vi "Scan Module.vi"(9 "Init state":T1=enum."Init(GPU FFT)", 11 "Error In":errorcluster, 12 "Start Acquire?":bool) -> (4 "Finished?":bool, 15 "Error Out":errorcluster)   [LabVIEW 2018]
uses:
  Controls/Go Scan Actions.ctl
  Controls/Queue Manager Actions.ctl
  Controls/FGV Actions.ctl
  Controls/Set Get Controls.ctl
  Hardware Mfg/Thorlabs Translation Stages/Controls/Motion Translation Module Control2.ctl
  Tile naming actions.ctl
  Controls/scan status.ctl
  Hardware Mfg/AlazarTech SDK/Controls/Alazar Engine Actions.ctl
  type defines/Pause action.ctl
  Controls/file variable action.ctl
  Controls/vibratome3 control.ctl
  Controls/Save Bline to Mem Control.ctl
  Hardware Mfg/Thorlabs Translation Stages/Controls/Motion Translation Module Control.ctl
panel:
  in  "No Slice?":bool
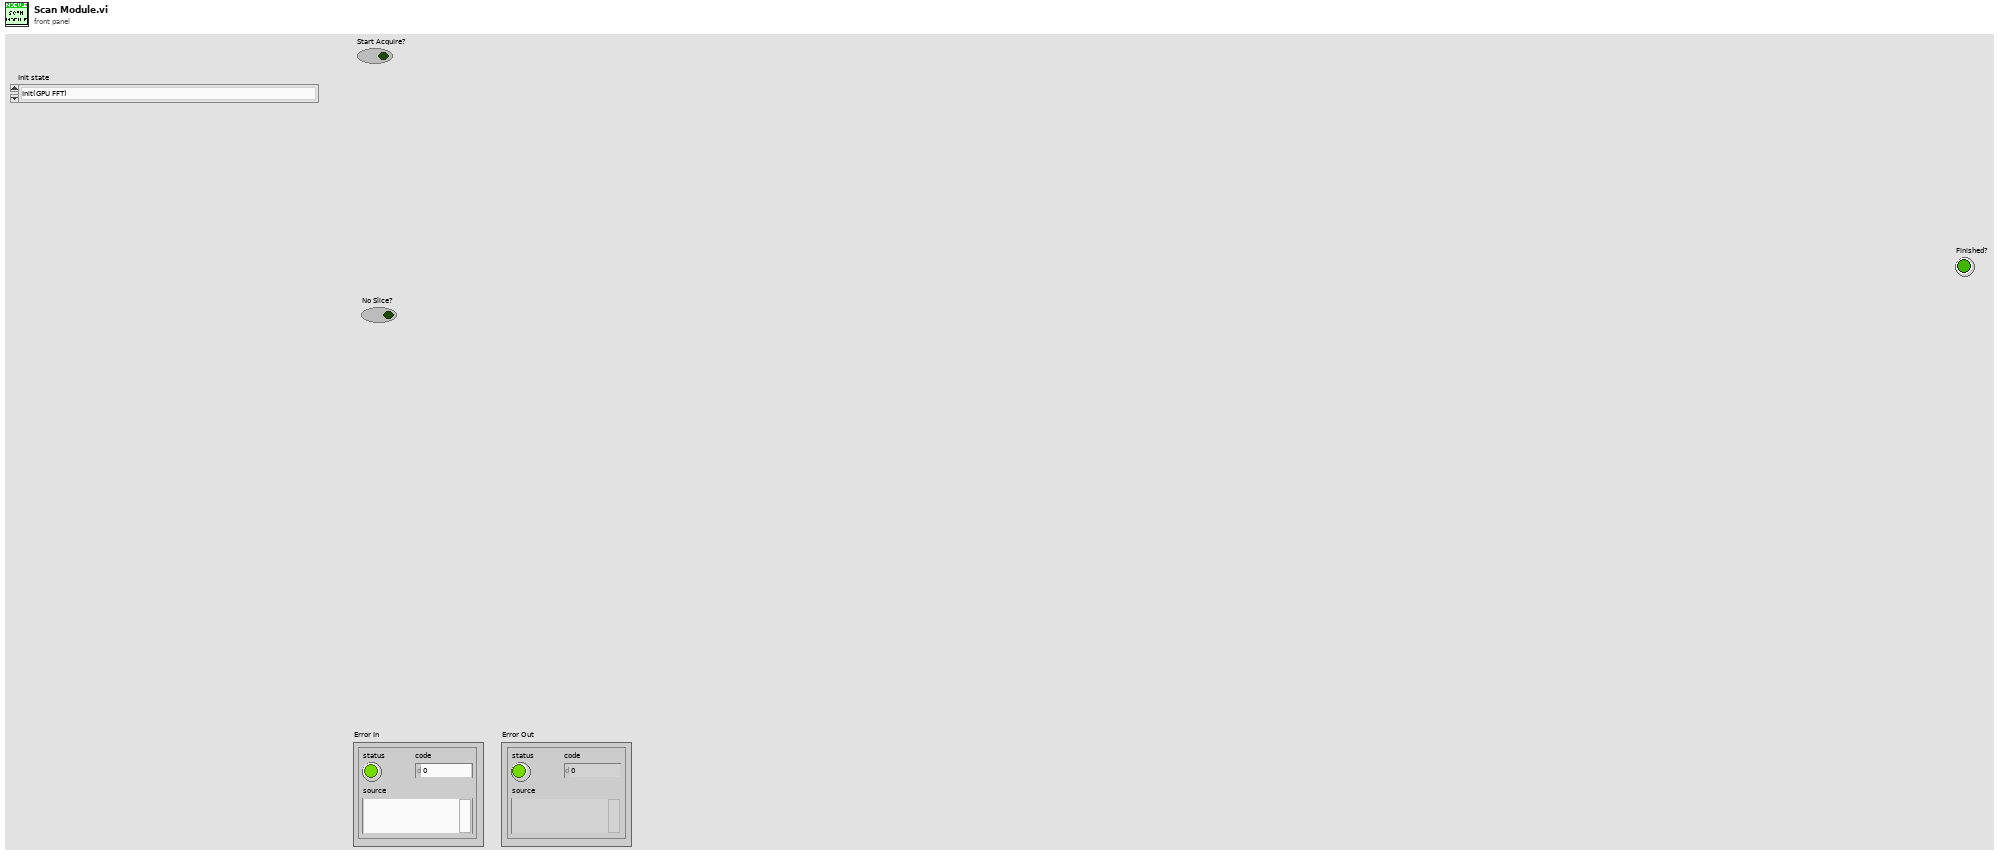
[diagram p1: front panel]
types:
  T1 = typedef "Go Scan Actions.ctl" = enum16{"Init(ThorOCT Spatial)", "Init(ThorOCT Spectral)", "Init(GPU FFT)", "Init(Alazar FFT)", "Init Scan Head(ThorOCT Spectral)", "Init Scan Head(ThorOCT Spatial)", "Init Scan Head", "Init Table Stage", "Init Vibratome", "Generate Mosaic", "Generate Z Position", "Go to Image Z", "Go Image Home", "Go Mosaic", "Acquire Image(ThorOCT Spatial)", "Acquire Image(ThorOCT Spectral)", "Acquire Image(GPU FFT)", "Acquire Image(Alazar FFT)", "Go Vibratome", "Slice", "Finished(ThorOCT)", "Finished", "Init(Alazar Spectral)", "Go Vibratome3"}
  T2 = typedef "Queue Manager Actions.ctl" = enum16{"Init", "Enqueue", "Enqueue All", "Preview Queue", "Dequeue", "Get Status", "Flush Queue", "Flush All Queues", "Release All Queues", "Release Queue", "Enqueue at Opposite End"}
  T3 = typedef "FGV Actions.ctl" = enum16{"Init", "Set", "Get", "Clear"}
  T4 = typedef "Motion Translation Module Control2.ctl" = enum16{"Init", "Home", "Status", "Velocity/Accel", "Position", "Jog", "Stop", "Uninit", "Enable", "Disable"}
  T5 = typedef "Set Get Controls.ctl" = enum16{"Set", "Get"}
  T6 = typedef "Motion Translation Module Control.ctl" = enum16{"Init", "Home", "Status", "Velocity/Accel", "Position", "Jog", "Stop", "Uninit", "Enable", "Disable"}
  T7 = typedef "Tile naming actions.ctl" = enum16{"Export", "Increment", "Total tile num", "Init"}
  T8 = typedef "scan status.ctl" = enum16{"Complete Scan(ThorOCT)", "Complete Scan(PSOCT)", "Start(ThorOCT Spatial)", "Start(ThorOCT Spectral)", "Start(GPU FFT)", "Start(Alazar FFT)", "Scan(ThorOCT Spatial)", "Scan(ThorOCT Spectral)", "Scan(GPU FFT)", "Scan(Alazar FFT)", "Finish Scan(ThorOCT)", "Finish Scan(PSOCT)", "Scan(simulate)", "Start(ROI)"}
  T9 = typedef "Alazar Engine Actions.ctl" = enum16{"Init", "Config Clock", "Config Ch", "Config Trig", "Config Non-FFT Acq.", "Non-FFT Acquire", "start acquire", "Config Acq.", "Acquire", "UnInit"}
  T10 = enum16{"Configure channels", "Write Scan Pattern", "Start Galvo Task", "Is Task Done?", "Stop Galvo", "Uninit", "Init: Calc scan pattern"}
  T11 = typedef "Pause action.ctl" = enum16{"Init", "get", "set"}
  T12 = typedef "file variable action.ctl" = enum16{"File name", "X stage", "Y stage", "Slice plane", "Image plane", "time", "output", "Init", "Memory Usage", "Disk full Space", "Disk free space"}
  T13 = typedef "vibratome3 control.ctl" = enum16{"Init", "Configure channel", "Write waveform", "Start", "Stop", "Finish?", "Uninit"}
  T14 = typedef "Save Bline to Mem Control.ctl" = enum16{"Output data", "Save(ThorOCT)", "Save(PSOCT)", "FFT and Save", "Uninit", "PSOCT Spectral buffer Set", "PSOCT Spatial buffer Set", "PSOCT Spectral buffer Init", "PSOCT Spatial buffer Init", "ThorOCT Spectral buffer Init", "ThorOCT Spatial buffer Init", "ThorOCT Spectral buffer Set", "ThorOCT Spatial buffer Set", "ThorOCT Spectral Save", "Alazar Spectral Save", "PSOCT save all"}
  T15 = typedef "ScanType.ctl" = enum16{"Single Frame", "Continuous Frame", "ROI Line", "Vibratome", "Mosaic", "Mosaic + Slice"}
  T16 = typedef "System Parameters.ctl" = cluster{"Optical Parameters":T17, "Vibratome":T18, "Table Stages":T19, "Imaging Parameter":T22, "Galvo HW Parameters":cluster{"Analog Out Channel":tag, "Min Voltage":dbl, "Max Voltage":dbl, "Pixel Clock Source":tag, "Sample Rate":dbl, "Line Clock Out Ch":tag}, "Alazar parameters":T24, "Mosaic Paramter":cluster{"X Axis":cluster{"Start [mm]":dbl, "Steps [pts]":dbl, "End [mm]":dbl}, "Y Axis":cluster{"Start [mm]":dbl, "Steps [pts]":dbl, "End [mm]":dbl}, "Scan Pattern":enum16{"Uni-directional", "Bi-Directional", "Spiral Out", "Spiral In"}, "Overlap Options":cluster{"Overlap Type":enum16{"No Overlap", "X Only", "Y Only", "X and Y"}, "Percent Overlap":u8, "Justify":enum16{"Start", "Center", "End"}}}, "Manual Controls":T31, "Vibratome Axis":T34}
  T17 = typedef "Optical Parameters.ctl" = cluster{"Obj. Focal Length [mm]":dbl, "Scan Lens EFL[mm]":dbl, "Tube Lens EFL[mm]":dbl, "Galvo V Range (+/-)":dbl, "Galvo Max Half Angle [Deg]":dbl, "Max Galvo Range[%]":dbl}
  T18 = typedef "Vibratome Parameters.ctl" = cluster{"Z Bottom [mm]":dbl, "Pre Cut Dwell [s]":dbl, "Blade Frequency [RPM]":u16, "Slice Speed [mm/s]":dbl, "Post Cut Dwell [s]":dbl, "Ramp Time [s]":dbl, "Start X [mm]":dbl, "Start Y [mm]":dbl, "Slice Length [mm]":dbl, "Slice Axis":enum16{"X Axis", "Y Axis", "Z Axis"}, "Controller VISA Ref":refnum<visa-resource-name>, "Blade Frequency [Hz]":u16, "Analog Out Channel":tag, "Pixel Clock Source":tag}
  T19 = typedef "Translation Stage Parameters.ctl" = cluster{"X Stage":T20, "Y Stage":T20, "Z Stage":T20}
  T20 = typedef "Translation Stage Cluster.ctl" = cluster{"Position":dbl, "Is.Enabled?":bool, "Is.Connected?":bool, "Device SN":string, "AccelerationMaximum":dbl, "VelocityMaximum":dbl, "Acceleration":dbl, "Velocity":dbl, "waitTimeout (ms)":i32, "Model":T21, "Is.Homed?":bool, "MOVE":bool}
  T21 = typedef "Translation Stage Types.ctl" = enum16{"None", "Thorlabs LTS", "Thorlabs MLJ"}
  T22 = typedef "Imaging Parameters.ctl" = cluster{"Raster Scan Direction":T23, "Pixel Dwell Time [Clock Cycles]":u16, "Flyback Time [Clock Cycles]":u16, "XY Center [um]":cluster{"X":dbl, "Y":dbl}, "Pixel Step Size [um] X":dbl, "XY Image Size":enum16{"32 x 32", "64 x 64", "128 x 128", "256 x 256", "512 x 512", "1024 x 1024", "2048 x 2048"}, "Custom":bool, "Custom Size":cluster{"X":u16, "Y":u16}, "Line Averages":u8, "Pixel Step Size [um] Y":dbl}
  T23 = typedef "Scan Direction.ctl" = enum16{"Uni Directional", "Bi Directional", "None"}
  T24 = typedef "Alazar parameters.ctl" = cluster{"Trigger Settings":cluster{"General Trigger Settings":T25, "Trigger Engine 1":T26, "Trigger Engine 2":T26}, "Device ID":T27, "Ch A Input Control":T28, "Ch B Input Control":T28, "Acq Settings":T29, "Capture Clock":T30}
  T25 = typedef "General Trigger Settings.ctl" = cluster{"Trigger Operation":u32, "Coupling ID":u32, "Range ID":u32, "Delay":u32, "Timeout Ticks":u32, "Mode":u32, "Parameter":u32}
  T26 = typedef "Trigger Engine Controls.ctl" = cluster{"Trigger Engine":u32, "Source":u32, "Slope":u32, "Level":u32}
  T27 = typedef "Alazar Device ID.ctl" = cluster{"System ID":u32, "Board ID":u32}
  T28 = typedef "Channel Input Controls.ctl" = cluster{"Channel":u8, "Coupling":u32, "Range":u32, "Impedance":u32}
  T29 = typedef "Alazar Acquisition Settings.ctl" = cluster{"Record Length":u32, "Offset":u32, "Records Per Buffer":u32, "Records Count (Records/Acq)":u32, "Window Type":u32, "Footer":u32, "Samples per record":u32, "Output Format":u32}
  T30 = typedef "Clock Controls.ctl" = cluster{"Sample Rate":u32, "Decimation":u32, "Source":u32, "Edge":u32}
  T31 = typedef "Manual Controls.ctl" = cluster{"Z0":dbl, "First image height":dbl, "Data Path":path, "Save parameters":T32, "Center Galvos":bool, "Acquisition mode":T33, "PSOCT Channel":u32, "Save":bool, "AIP rotation angle":dbl, "ret ds":bool, "Pause?":bool, "Outgoing Mail Server (SMTP)":string, "Email":string, "Password":string, "Carrier 1":enum16{"T-Mobile", "AT&T", "Verizon", "Sprint"}, "phone number 1":string, "Subject":string, "Message":string, "blocker position":enum16{"every two slices", "Nat slices", "None"}, "Carrier 2":enum16{"T-Mobile", "AT&T", "Verizon", "Sprint"}, "phone number 2":string}
  T32 = typedef "FFT parameters.ctl" = cluster{"start pixel":i32, "#pixels to save":i32}
  T33 = typedef "FFT mode.ctl" = enum16{"ThorOCT B line", "ThorOCT Spectral", "ThorOCT FFT", "Alazar B line", "Alazar FFT", "GPU FFT", "Alazar Spectral", "Simulation", "auto adjust focus", "Save all"}
  T34 = typedef "Vibratome Param.ctl" = cluster{"Start [mm](first cut height)":dbl, "slice thickness[um]":dbl, "#slice":u16, "image thickness(um)":dbl, "#images":u16, "30um?":bool}
  T35 = cluster{"X Axis":cluster{"Start [mm]":dbl, "Steps [pts]":dbl, "End [mm]":dbl}, "Y Axis":cluster{"Start [mm]":dbl, "Steps [pts]":dbl, "End [mm]":dbl}, "Scan Pattern":enum16{"Uni-directional", "Bi-Directional", "Spiral Out", "Spiral In"}, "Overlap Options":cluster{"Overlap Type":enum16{"No Overlap", "X Only", "Y Only", "X and Y"}, "Percent Overlap":u8, "Justify":enum16{"Start", "Center", "End"}}}
  T36 = cluster{"Start [mm]":dbl, "Steps [pts]":dbl, "End [mm]":dbl}
  T37 = cluster{"Overlap Type":enum16{"No Overlap", "X Only", "Y Only", "X and Y"}, "Percent Overlap":u8, "Justify":enum16{"Start", "Center", "End"}}
  T38 = enum16{"Uni-directional", "Bi-Directional", "Spiral Out", "Spiral In"}
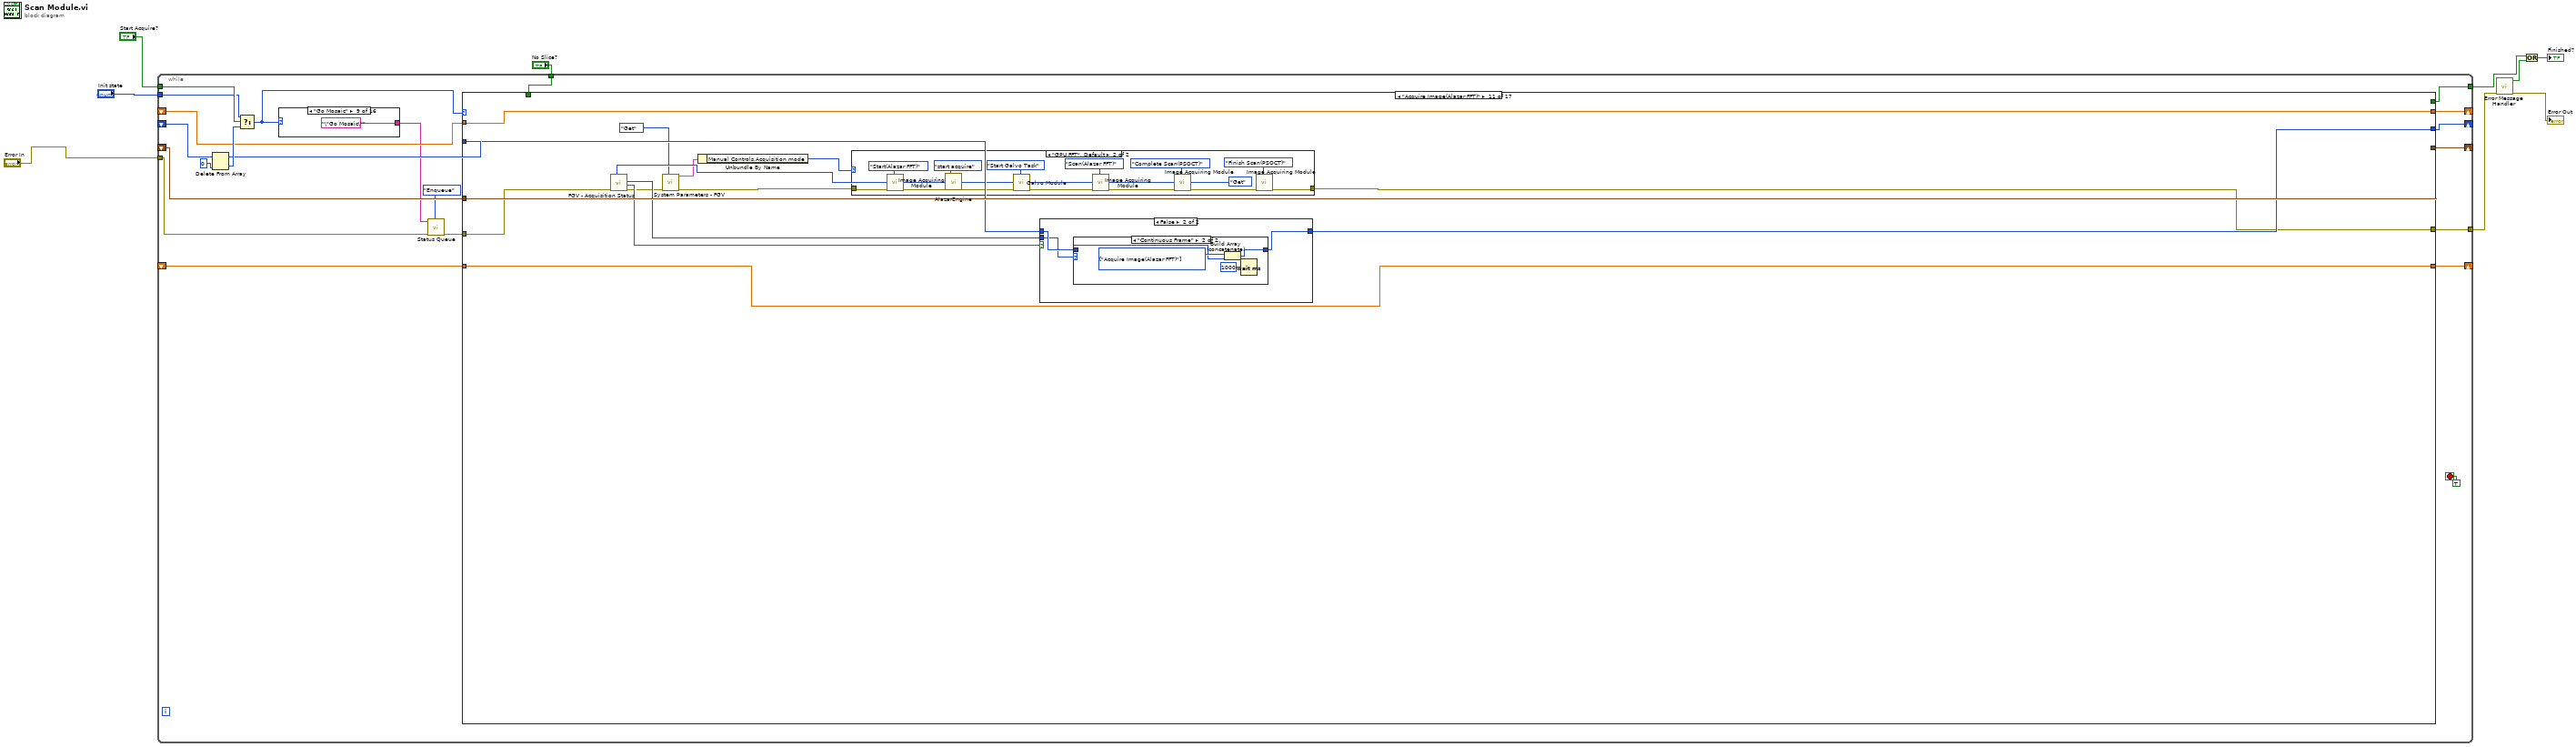
[diagram p0: block diagram]
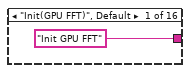
[diagram p2: hidden frame]
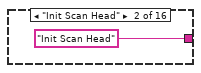
[diagram p3: hidden frame]
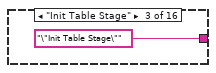
[diagram p4: hidden frame]
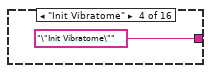
[diagram p5: hidden frame]
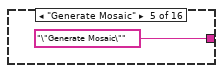
[diagram p6: hidden frame]
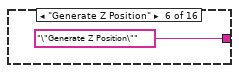
[diagram p7: hidden frame]
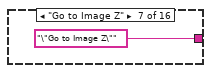
[diagram p8: hidden frame]
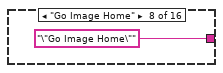
[diagram p9: hidden frame]
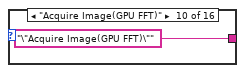
[diagram p10: hidden frame]
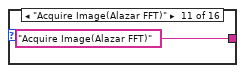
[diagram p11: hidden frame]
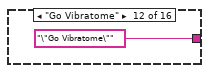
[diagram p12: hidden frame]
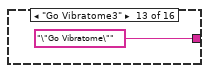
[diagram p13: hidden frame]
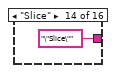
[diagram p14: hidden frame]
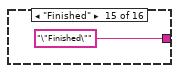
[diagram p15: hidden frame]
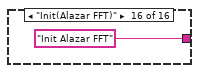
[diagram p16: hidden frame]
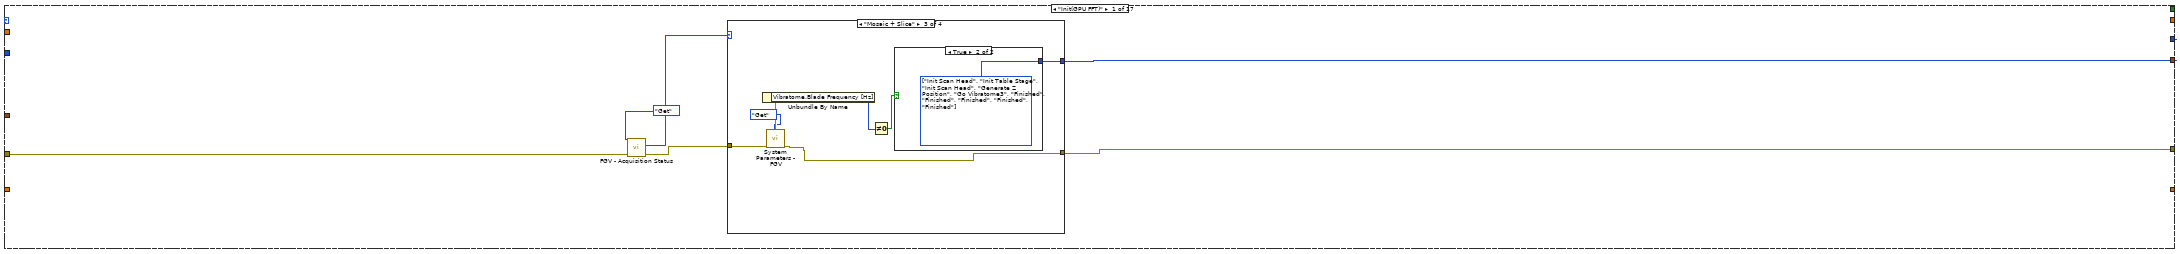
[diagram p17: hidden frame]
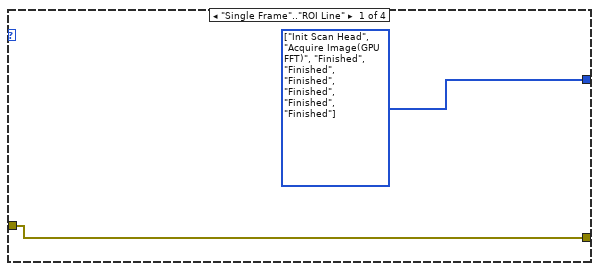
[diagram p18: hidden frame]
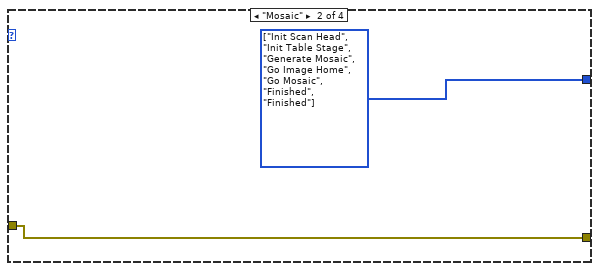
[diagram p19: hidden frame]
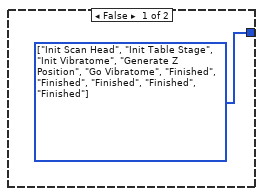
[diagram p20: hidden frame]
diagram:
  n1 = while {
    shift-right: [w25] -> _
    shift-left: _ -> [w30]
    tunnel: "Start Acquire?" -> [w26]
    shift-right: [w24] -> _
    shift-left: _ -> [w22]
    tunnel: "Error In" -> [w15]
    tunnel: [w23] -> w9
    tunnel: [w21] -> w6
    shift-right: [w19] -> _
    shift-left: _ -> [w17]
    shift-right: [w20] -> _
    shift-left: _ -> [w18]
    tunnel: "Init state" -> [w16]
    tunnel: "No Slice?" -> [w10]
    stop <- TRUE stop-if-true
    n2 = Delete From Array(array=w30, index=0) -> (deleted portion=w29:T1, array with subset deleted=w28:T1[])  [unwired: 1 in]
    n3 = Select(t=w16, s=w26, f=w29) -> (s? t:f=w13:T1)
    n4 = case shown="\"Go Mosaic\"" w13 {
      tunnel: ["Init GPU FFT" "Init Scan Head" "\"Init Table Stage\"" "\"Init Vibratome\"" "\"Generate Mosaic\"" "\"Generate Z Position\"" "\"Go to Image Z\"" "\"Go Image Home\"" "\"Go Mosaic\"" "\"Acquire Image(GPU FFT)\"" "Acquire Image(Alazar FFT)" "\"Go Vibratome\"" "\"Go Vibratome\"" "\"Slice\"" "\"Finished\"" "Init Alazar FFT"] -> w12
      frame "Init(GPU FFT)", Default {
      }
      frame "Init Scan Head" {
      }
      frame "Init Table Stage" {
      }
      frame "Init Vibratome" {
      }
      frame "Generate Mosaic" {
      }
      frame "Generate Z Position" {
      }
      frame "Go to Image Z" {
      }
      frame "Go Image Home" {
      }
      frame "Go Mosaic" {
      }
      frame "Acquire Image(GPU FFT)" {
      }
      frame "Acquire Image(Alazar FFT)" {
      }
      frame "Go Vibratome" {
      }
      frame "Go Vibratome3" {
      }
      frame "Slice" {
      }
      frame "Finished" {
      }
      frame "Init(Alazar FFT)" {
      }
    }
    n5 = call "Status Queue.vi"("Action"=Queue_Manager_Actions."Enqueue", "Error In"=w15, "Status Message [In]"=w12) -> ("Error Out"=w14:errorcluster)  [unwired: 7 in, 1 out]
    n6 = case shown="\"Acquire Image(Alazar FFT)\"" w13 {
      selector: w13 -> [_ _ _ _ _ _ _ _ _ _ _ _ w388 _ _ _ _]
      tunnel: [w52 w79 w88 w132 w137 w147 w193 w218 w227 w258 w313 w355 w394 w484 w720 w1089 _] -> w25
      tunnel: w28 -> [_ _ _ w132 w137 w147 w193 w218 w227 w259 w316 w356 w386 w486 w722 w1091 _]
      tunnel: [_ _ _ w133 w138 w148 w194 w208 w228 w266 w319 w360 w396 w487 w723 w1092 _] -> w24
      tunnel: w22 -> [_ _ _ w133 w138 w148 w194 _ w228 w266 w319 w360 w387 w487 w723 w1092 _]
      tunnel: [w48 w76 w85 w116 w134 w146 w190 w202 w224 w265 w312 w343 w395 w485 w721 w1090 w1112] -> w23
      tunnel: [_ _ _ _ _ _ _ _ _ _ _ _ _ _ _ w1085 TRUE] -> w21
      tunnel: [_ _ _ w130 w135 w144 w192 w212 w226 w264 w318 w358 w391 w480 w716 w1084 _] -> w20
      tunnel: [_ _ _ w124 w136 w145 w191 w211 w225 w262 w317 w357 w390 w479 w715 w1087 _] -> w19
      tunnel: w18 -> [_ _ _ _ w135 w144 w192 w212 w226 w264 w318 w358 w391 w478 w714 w1084 _]
      tunnel: w17 -> [_ _ _ _ w136 w145 w191 w211 w225 w260 w317 w357 w390 w479 w715 w1087 _]
      tunnel: w14 -> [w50 w77 w87 w117 w134 w142 w189 w205 w222 w263 w310 w353 w385 w483 w719 w1088 w1115]
      tunnel: w10 -> [_ _ _ _ _ _ _ _ _ _ _ _ _ w477 w713 _ _]
      frame "Init(GPU FFT)" {
        n7 = call "FGV - Acquisition Status.vi"("Actions"=FGV_Actions."Get", "Error In"=w50) -> ("Error Out"=w49:errorcluster, "Scan Type [Out]"=w51:T15)  [unwired: 6 in, 2 out]
        n8 = case shown="\"Mosaic + Slice\"" w51 {
          tunnel: [w55 w57 w64 w73] -> w52
          tunnel: w49 -> [w54 w56 w60 w72]
          tunnel: [w54 w56 w59 w71] -> w48
          frame "Single Frame".."ROI Line" {
            w55 = T1[] [enum."Init Scan Head", enum."Acquire Image(GPU FFT)", enum."Finished", enum."Finished", enum."Finished", enum."Finished", enum."Finished", enum."Finished"] items=["Init(ThorOCT Spatial)", "Init(ThorOCT Spectral)", "Init(GPU FFT)", "Init(Alazar FFT)", "Init Scan Head(ThorOCT Spectral)", "Init Scan Head(ThorOCT Spatial)", "Init Scan Head", "Init Table Stage", "Init Vibratome", "Generate Mosaic", "Generate Z Position", "Go to Image Z", "Go Image Home", "Go Mosaic", "Acquire Image(ThorOCT Spatial)", "Acquire Image(ThorOCT Spectral)", "Acquire Image(GPU FFT)", "Acquire Image(Alazar FFT)", "Go Vibratome", "Slice", "Finished(ThorOCT)", "Finished", "Init(Alazar Spectral)", "Go Vibratome3"]
          }
          frame "Mosaic" {
            w57 = T1[] [enum."Init Scan Head", enum."Init Table Stage", enum."Generate Mosaic", enum."Go Image Home", enum."Go Mosaic", enum."Finished", enum."Finished"] items=["Init(ThorOCT Spatial)", "Init(ThorOCT Spectral)", "Init(GPU FFT)", "Init(Alazar FFT)", "Init Scan Head(ThorOCT Spectral)", "Init Scan Head(ThorOCT Spatial)", "Init Scan Head", "Init Table Stage", "Init Vibratome", "Generate Mosaic", "Generate Z Position", "Go to Image Z", "Go Image Home", "Go Mosaic", "Acquire Image(ThorOCT Spatial)", "Acquire Image(ThorOCT Spectral)", "Acquire Image(GPU FFT)", "Acquire Image(Alazar FFT)", "Go Vibratome", "Slice", "Finished(ThorOCT)", "Finished", "Init(Alazar Spectral)", "Go Vibratome3"]
          }
          frame "Mosaic + Slice" {
            n9 = call "System Parameters - FGV.vi"("Actions"=FGV_Actions."Get", "Error In"=w60) -> ("Error Out"=w59:errorcluster, "System Parameters [Out]"=w62:T16)  [unwired: 8 in]
            n10 = Unbundle By Name(w62) -> ("Vibratome.Blade Frequency [Hz]"=w63:u16)
            n11 = Not Equal To 0?(x=w63) -> (x != 0?=w58:bool)
            n12 = case shown="True" w58 {
              tunnel: [w65 w66] -> w64
              frame False {
                w65 = T1[] [enum."Init Scan Head", enum."Init Table Stage", enum."Init Vibratome", enum."Generate Z Position", enum."Go Vibratome", enum."Finished", enum."Finished", enum."Finished", enum."Finished", enum."Finished"] items=["Init(ThorOCT Spatial)", "Init(ThorOCT Spectral)", "Init(GPU FFT)", "Init(Alazar FFT)", "Init Scan Head(ThorOCT Spectral)", "Init Scan Head(ThorOCT Spatial)", "Init Scan Head", "Init Table Stage", "Init Vibratome", "Generate Mosaic", "Generate Z Position", "Go to Image Z", "Go Image Home", "Go Mosaic", "Acquire Image(ThorOCT Spatial)", "Acquire Image(ThorOCT Spectral)", "Acquire Image(GPU FFT)", "Acquire Image(Alazar FFT)", "Go Vibratome", "Slice", "Finished(ThorOCT)", "Finished", "Init(Alazar Spectral)", "Go Vibratome3"]
              }
              frame True {
                w66 = T1[] [enum."Init Scan Head", enum."Init Table Stage", enum."Init Scan Head", enum."Generate Z Position", enum."Go Vibratome3", enum."Finished", enum."Finished", enum."Finished", enum."Finished", enum."Finished"] items=["Init(ThorOCT Spatial)", "Init(ThorOCT Spectral)", "Init(GPU FFT)", "Init(Alazar FFT)", "Init Scan Head(ThorOCT Spectral)", "Init Scan Head(ThorOCT Spatial)", "Init Scan Head", "Init Table Stage", "Init Vibratome", "Generate Mosaic", "Generate Z Position", "Go to Image Z", "Go Image Home", "Go Mosaic", "Acquire Image(ThorOCT Spatial)", "Acquire Image(ThorOCT Spectral)", "Acquire Image(GPU FFT)", "Acquire Image(Alazar FFT)", "Go Vibratome", "Slice", "Finished(ThorOCT)", "Finished", "Init(Alazar Spectral)", "Go Vibratome3"]
              }
            }
          }
          frame "Vibratome" {
            n13 = call "System Parameters - FGV.vi"("Actions"=FGV_Actions."Get", "Error In"=w72) -> ("Error Out"=w71:errorcluster, "System Parameters [Out]"=w69:T16)  [unwired: 8 in]
            n14 = Unbundle By Name(w69) -> ("Vibratome.Blade Frequency [Hz]"=w68:u16)
            n15 = Not Equal To 0?(x=w68) -> (x != 0?=w67:bool)
            n16 = case shown="True" w67 {
              tunnel: [w74 w75] -> w73
              frame False {
                w74 = T1[] [enum."Init Table Stage", enum."Init Vibratome", enum."Slice", enum."Finished", enum."Finished"] items=["Init(ThorOCT Spatial)", "Init(ThorOCT Spectral)", "Init(GPU FFT)", "Init(Alazar FFT)", "Init Scan Head(ThorOCT Spectral)", "Init Scan Head(ThorOCT Spatial)", "Init Scan Head", "Init Table Stage", "Init Vibratome", "Generate Mosaic", "Generate Z Position", "Go to Image Z", "Go Image Home", "Go Mosaic", "Acquire Image(ThorOCT Spatial)", "Acquire Image(ThorOCT Spectral)", "Acquire Image(GPU FFT)", "Acquire Image(Alazar FFT)", "Go Vibratome", "Slice", "Finished(ThorOCT)", "Finished", "Init(Alazar Spectral)", "Go Vibratome3"]
              }
              frame True {
                w75 = T1[] [enum."Init Table Stage", enum."Init Scan Head", enum."Slice", enum."Finished", enum."Finished"] items=["Init(ThorOCT Spatial)", "Init(ThorOCT Spectral)", "Init(GPU FFT)", "Init(Alazar FFT)", "Init Scan Head(ThorOCT Spectral)", "Init Scan Head(ThorOCT Spatial)", "Init Scan Head", "Init Table Stage", "Init Vibratome", "Generate Mosaic", "Generate Z Position", "Go to Image Z", "Go Image Home", "Go Mosaic", "Acquire Image(ThorOCT Spatial)", "Acquire Image(ThorOCT Spectral)", "Acquire Image(GPU FFT)", "Acquire Image(Alazar FFT)", "Go Vibratome", "Slice", "Finished(ThorOCT)", "Finished", "Init(Alazar Spectral)", "Go Vibratome3"]
              }
            }
          }
        }
      }
      frame "Init(Alazar Spectral)" {
        n17 = call "FGV - Acquisition Status.vi"("Actions"=FGV_Actions."Get", "Error In"=w77) -> ("Error Out"=w76:errorcluster, "Scan Type [Out]"=w78:T15)  [unwired: 6 in, 2 out]
        n18 = case shown="\"Mosaic + Slice\"" w78 {
          tunnel: [w81 w82 w83 w84] -> w79
          frame "Single Frame".."ROI Line" {
            w81 = T1[] [enum."Init Scan Head", enum."Init Scan Head", enum."Acquire Image(GPU FFT)", enum."Finished", enum."Acquire Image(GPU FFT)", enum."Finished", enum."Acquire Image(GPU FFT)", enum."Finished"] items=["Init(ThorOCT Spatial)", "Init(ThorOCT Spectral)", "Init(GPU FFT)", "Init(Alazar FFT)", "Init Scan Head(ThorOCT Spectral)", "Init Scan Head(ThorOCT Spatial)", "Init Scan Head", "Init Table Stage", "Init Vibratome", "Generate Mosaic", "Generate Z Position", "Go to Image Z", "Go Image Home", "Go Mosaic", "Acquire Image(ThorOCT Spatial)", "Acquire Image(ThorOCT Spectral)", "Acquire Image(GPU FFT)", "Acquire Image(Alazar FFT)", "Go Vibratome", "Slice", "Finished(ThorOCT)", "Finished", "Init(Alazar Spectral)", "Go Vibratome3"]
          }
          frame "Mosaic" {
            w82 = T1[] [enum."Init Scan Head", enum."Init Table Stage", enum."Generate Mosaic", enum."Go Image Home", enum."Go Mosaic", enum."Finished", enum."Finished"] items=["Init(ThorOCT Spatial)", "Init(ThorOCT Spectral)", "Init(GPU FFT)", "Init(Alazar FFT)", "Init Scan Head(ThorOCT Spectral)", "Init Scan Head(ThorOCT Spatial)", "Init Scan Head", "Init Table Stage", "Init Vibratome", "Generate Mosaic", "Generate Z Position", "Go to Image Z", "Go Image Home", "Go Mosaic", "Acquire Image(ThorOCT Spatial)", "Acquire Image(ThorOCT Spectral)", "Acquire Image(GPU FFT)", "Acquire Image(Alazar FFT)", "Go Vibratome", "Slice", "Finished(ThorOCT)", "Finished", "Init(Alazar Spectral)", "Go Vibratome3"]
          }
          frame "Mosaic + Slice" {
            w83 = T1[] [enum."Init Scan Head", enum."Init Table Stage", enum."Init Vibratome", enum."Generate Z Position", enum."Go Vibratome", enum."Finished", enum."Finished", enum."Finished", enum."Finished", enum."Finished"] items=["Init(ThorOCT Spatial)", "Init(ThorOCT Spectral)", "Init(GPU FFT)", "Init(Alazar FFT)", "Init Scan Head(ThorOCT Spectral)", "Init Scan Head(ThorOCT Spatial)", "Init Scan Head", "Init Table Stage", "Init Vibratome", "Generate Mosaic", "Generate Z Position", "Go to Image Z", "Go Image Home", "Go Mosaic", "Acquire Image(ThorOCT Spatial)", "Acquire Image(ThorOCT Spectral)", "Acquire Image(GPU FFT)", "Acquire Image(Alazar FFT)", "Go Vibratome", "Slice", "Finished(ThorOCT)", "Finished", "Init(Alazar Spectral)", "Go Vibratome3"]
          }
          frame "Vibratome" {
            w84 = T1[] [enum."Init Table Stage", enum."Init Vibratome", enum."Slice", enum."Finished", enum."Finished"] items=["Init(ThorOCT Spatial)", "Init(ThorOCT Spectral)", "Init(GPU FFT)", "Init(Alazar FFT)", "Init Scan Head(ThorOCT Spectral)", "Init Scan Head(ThorOCT Spatial)", "Init Scan Head", "Init Table Stage", "Init Vibratome", "Generate Mosaic", "Generate Z Position", "Go to Image Z", "Go Image Home", "Go Mosaic", "Acquire Image(ThorOCT Spatial)", "Acquire Image(ThorOCT Spectral)", "Acquire Image(GPU FFT)", "Acquire Image(Alazar FFT)", "Go Vibratome", "Slice", "Finished(ThorOCT)", "Finished", "Init(Alazar Spectral)", "Go Vibratome3"]
          }
        }
      }
      frame "Init(Alazar FFT)" {
        n19 = call "FGV - Acquisition Status.vi"("Actions"=FGV_Actions."Get", "Error In"=w87) -> ("Error Out"=w86:errorcluster, "Scan Type [Out]"=w89:T15)  [unwired: 6 in, 2 out]
        n20 = case shown="\"Mosaic + Slice\"" w89 {
          tunnel: [w92 w94 w96 w103 w112] -> w88
          tunnel: w86 -> [w91 w93 w95 w99 w108]
          tunnel: [w91 w93 w95 w97 w107] -> w85
          frame "Single Frame", Default {
            w92 = T1[] [enum."Init Scan Head", enum."Acquire Image(Alazar FFT)", enum."Finished", enum."Finished", enum."Acquire Image(Alazar FFT)", enum."Finished", enum."Acquire Image(Alazar FFT)", enum."Finished"] items=["Init(ThorOCT Spatial)", "Init(ThorOCT Spectral)", "Init(GPU FFT)", "Init(Alazar FFT)", "Init Scan Head(ThorOCT Spectral)", "Init Scan Head(ThorOCT Spatial)", "Init Scan Head", "Init Table Stage", "Init Vibratome", "Generate Mosaic", "Generate Z Position", "Go to Image Z", "Go Image Home", "Go Mosaic", "Acquire Image(ThorOCT Spatial)", "Acquire Image(ThorOCT Spectral)", "Acquire Image(GPU FFT)", "Acquire Image(Alazar FFT)", "Go Vibratome", "Slice", "Finished(ThorOCT)", "Finished", "Init(Alazar Spectral)", "Go Vibratome3"]
          }
          frame "Continuous Frame" {
            w94 = T1[] [enum."Init Scan Head", enum."Acquire Image(Alazar FFT)", enum."Finished", enum."Finished", enum."Acquire Image(Alazar FFT)", enum."Finished", enum."Acquire Image(Alazar FFT)", enum."Finished"] items=["Init(ThorOCT Spatial)", "Init(ThorOCT Spectral)", "Init(GPU FFT)", "Init(Alazar FFT)", "Init Scan Head(ThorOCT Spectral)", "Init Scan Head(ThorOCT Spatial)", "Init Scan Head", "Init Table Stage", "Init Vibratome", "Generate Mosaic", "Generate Z Position", "Go to Image Z", "Go Image Home", "Go Mosaic", "Acquire Image(ThorOCT Spatial)", "Acquire Image(ThorOCT Spectral)", "Acquire Image(GPU FFT)", "Acquire Image(Alazar FFT)", "Go Vibratome", "Slice", "Finished(ThorOCT)", "Finished", "Init(Alazar Spectral)", "Go Vibratome3"]
          }
          frame "Mosaic" {
            w96 = T1[] [enum."Init Scan Head", enum."Init Table Stage", enum."Generate Mosaic", enum."Go Image Home", enum."Go Mosaic", enum."Finished", enum."Finished"] items=["Init(ThorOCT Spatial)", "Init(ThorOCT Spectral)", "Init(GPU FFT)", "Init(Alazar FFT)", "Init Scan Head(ThorOCT Spectral)", "Init Scan Head(ThorOCT Spatial)", "Init Scan Head", "Init Table Stage", "Init Vibratome", "Generate Mosaic", "Generate Z Position", "Go to Image Z", "Go Image Home", "Go Mosaic", "Acquire Image(ThorOCT Spatial)", "Acquire Image(ThorOCT Spectral)", "Acquire Image(GPU FFT)", "Acquire Image(Alazar FFT)", "Go Vibratome", "Slice", "Finished(ThorOCT)", "Finished", "Init(Alazar Spectral)", "Go Vibratome3"]
          }
          frame "Mosaic + Slice" {
            n21 = call "System Parameters - FGV.vi"("Actions"=FGV_Actions."Get", "Error In"=w99) -> ("Error Out"=w97:errorcluster, "System Parameters [Out]"=w101:T16)  [unwired: 8 in]
            n22 = Unbundle By Name(w101) -> ("Vibratome.Blade Frequency [Hz]"=w102:u16)
            n23 = Not Equal To 0?(x=w102) -> (x != 0?=w98:bool)
            n24 = case shown="False" w98 {
              tunnel: [w104 w105] -> w103
              frame False {
                w104 = T1[] [enum."Init Scan Head", enum."Init Table Stage", enum."Init Vibratome", enum."Generate Z Position", enum."Go Vibratome", enum."Finished"] items=["Init(ThorOCT Spatial)", "Init(ThorOCT Spectral)", "Init(GPU FFT)", "Init(Alazar FFT)", "Init Scan Head(ThorOCT Spectral)", "Init Scan Head(ThorOCT Spatial)", "Init Scan Head", "Init Table Stage", "Init Vibratome", "Generate Mosaic", "Generate Z Position", "Go to Image Z", "Go Image Home", "Go Mosaic", "Acquire Image(ThorOCT Spatial)", "Acquire Image(ThorOCT Spectral)", "Acquire Image(GPU FFT)", "Acquire Image(Alazar FFT)", "Go Vibratome", "Slice", "Finished(ThorOCT)", "Finished", "Init(Alazar Spectral)", "Go Vibratome3"]
              }
              frame True {
                w105 = T1[] [enum."Init Scan Head", enum."Init Table Stage", enum."Init Scan Head", enum."Generate Z Position", enum."Go Vibratome3", enum."Finished"] items=["Init(ThorOCT Spatial)", "Init(ThorOCT Spectral)", "Init(GPU FFT)", "Init(Alazar FFT)", "Init Scan Head(ThorOCT Spectral)", "Init Scan Head(ThorOCT Spatial)", "Init Scan Head", "Init Table Stage", "Init Vibratome", "Generate Mosaic", "Generate Z Position", "Go to Image Z", "Go Image Home", "Go Mosaic", "Acquire Image(ThorOCT Spatial)", "Acquire Image(ThorOCT Spectral)", "Acquire Image(GPU FFT)", "Acquire Image(Alazar FFT)", "Go Vibratome", "Slice", "Finished(ThorOCT)", "Finished", "Init(Alazar Spectral)", "Go Vibratome3"]
              }
            }
          }
          frame "Vibratome" {
            n25 = call "System Parameters - FGV.vi"("Actions"=FGV_Actions."Get", "Error In"=w108) -> ("Error Out"=w107:errorcluster, "System Parameters [Out]"=w110:T16)  [unwired: 8 in]
            n26 = Unbundle By Name(w110) -> ("Vibratome.Blade Frequency [Hz]"=w111:u16)
            n27 = Not Equal To 0?(x=w111) -> (x != 0?=w106:bool)
            n28 = case shown="True" w106 {
              tunnel: [w113 w114] -> w112
              frame False {
                w113 = T1[] [enum."Init Table Stage", enum."Init Vibratome", enum."Slice", enum."Finished", enum."Finished"] items=["Init(ThorOCT Spatial)", "Init(ThorOCT Spectral)", "Init(GPU FFT)", "Init(Alazar FFT)", "Init Scan Head(ThorOCT Spectral)", "Init Scan Head(ThorOCT Spatial)", "Init Scan Head", "Init Table Stage", "Init Vibratome", "Generate Mosaic", "Generate Z Position", "Go to Image Z", "Go Image Home", "Go Mosaic", "Acquire Image(ThorOCT Spatial)", "Acquire Image(ThorOCT Spectral)", "Acquire Image(GPU FFT)", "Acquire Image(Alazar FFT)", "Go Vibratome", "Slice", "Finished(ThorOCT)", "Finished", "Init(Alazar Spectral)", "Go Vibratome3"]
              }
              frame True {
                w114 = T1[] [enum."Init Table Stage", enum."Init Scan Head", enum."Slice", enum."Finished", enum."Finished"] items=["Init(ThorOCT Spatial)", "Init(ThorOCT Spectral)", "Init(GPU FFT)", "Init(Alazar FFT)", "Init Scan Head(ThorOCT Spectral)", "Init Scan Head(ThorOCT Spatial)", "Init Scan Head", "Init Table Stage", "Init Vibratome", "Generate Mosaic", "Generate Z Position", "Go to Image Z", "Go Image Home", "Go Mosaic", "Acquire Image(ThorOCT Spatial)", "Acquire Image(ThorOCT Spectral)", "Acquire Image(GPU FFT)", "Acquire Image(Alazar FFT)", "Go Vibratome", "Slice", "Finished(ThorOCT)", "Finished", "Init(Alazar Spectral)", "Go Vibratome3"]
              }
            }
          }
        }
      }
      frame "Generate Z Position" {
        w123 = 0.0
        w127 = 0.0 ("y")
        n29 = call "System Parameters - FGV.vi"("Actions"=FGV_Actions."Get", "Error In"=w117) -> ("Error Out"=w116:errorcluster, "System Parameters [Out]"=w115:T16)  [unwired: 8 in]
        n30 = Unbundle By Name(w115) -> ("Vibratome Axis"=w131:T34)
        n31 = Unbundle By Name(w131) -> ("Start [mm](first cut height)"=w129:dbl, "slice thickness[um]"=w128:dbl, "#slice"=w126:u16)
        n32 = Unbundle By Name(w115) -> ("Manual Controls.First image height"=w119:dbl)
        n33 = call "Generate Z stage Position Aarray.vi"("#rep1"=w126, "#rep2"=w127, "thickness2"=w127, "Start Z"=w129, "thickness1"=w128) -> ("Array"=w130:dbl[])  [unwired: 6 in]
        n34 = Unbundle By Name(w131) -> ("image thickness(um)"=w120:dbl, "#images"=w125:u16)
        n35 = Multiply(x=w126, y=w125) -> (x*y=w122:u16)
        n36 = Decrement(x=w122) -> (x-1=w121:u16)
        n37 = call "Generate Z stage Position Aarray.vi"("#rep1"=w121, "#rep2"=w123, "thickness2"=w123, "Start Z"=w119, "thickness1"=w120) -> ("Array"=w124:dbl[])  [unwired: 6 in]
      }
      frame "Init Scan Head" {
      }
      frame "Init Table Stage" {
        n38 = call "System Parameters - FGV.vi"("Actions"=FGV_Actions."Get", "Error In"=w142) -> ("Error Out"=w141:errorcluster, "System Parameters [Out]"=w140:T16)  [unwired: 8 in]
        n39 = Unbundle By Name(w140) -> ("Manual Controls.Acquisition mode"=w139:T33)
        n40 = case shown="\"GPU FFT\", Default" w139 {
          tunnel: [w149 w157] -> w146
          tunnel: w141 -> [w149 w160]
          tunnel: w140 -> [_ w159]
          frame "Simulation" {
          }
          frame "GPU FFT", Default {
            n41 = Unbundle By Name(w159) -> ("Table Stages"=w156:T19)
            n42 = call "XYZ Table Stage Module.vi"("Set/Get"=Set_Get_Controls."Set", "Action"=Motion_Translation_Module_Control2."Init", "Error In"=w160, "Axis"=enum16{"X Axis", "Y Axis", "Z Axis"}."X Axis", "Table Stages"=w156) -> ("Error Out"=w177:errorcluster)  [unwired: 5 in, 1 out]
            n43 = call "XYZ Table Stage Module.vi"("Set/Get"=Set_Get_Controls."Set", "Action"=Motion_Translation_Module_Control2."Init", "Error In"=w177, "Axis"=enum16{"X Axis", "Y Axis", "Z Axis"}."Y Axis", "Table Stages"=w156) -> ("Error Out"=w172:errorcluster)  [unwired: 5 in, 1 out]
            n44 = call "XYZ Table Stage Module.vi"("Set/Get"=Set_Get_Controls."Set", "Action"=Motion_Translation_Module_Control2."Init", "Error In"=w172, "Axis"=enum16{"X Axis", "Y Axis", "Z Axis"}."Z Axis", "Table Stages"=w156) -> ("Error Out"=w161:errorcluster)  [unwired: 5 in, 1 out]
            n45 = call "XYZ Table Stage Module.vi"("Set/Get"=Set_Get_Controls."Set", "Action"=Motion_Translation_Module_Control2."Velocity/Accel", "Error In"=w161, "Axis"=enum16{"X Axis", "Y Axis", "Z Axis"}."X Axis", "Table Stages"=w156) -> ("Error Out"=w169:errorcluster)  [unwired: 5 in, 1 out]
            n46 = call "XYZ Table Stage Module.vi"("Set/Get"=Set_Get_Controls."Set", "Action"=Motion_Translation_Module_Control2."Velocity/Accel", "Error In"=w169, "Axis"=enum16{"X Axis", "Y Axis", "Z Axis"}."Y Axis", "Table Stages"=w156) -> ("Error Out"=w164:errorcluster)  [unwired: 5 in, 1 out]
            n47 = call "XYZ Table Stage Module.vi"("Set/Get"=Set_Get_Controls."Set", "Action"=Motion_Translation_Module_Control2."Velocity/Accel", "Error In"=w164, "Axis"=enum16{"X Axis", "Y Axis", "Z Axis"}."Z Axis", "Table Stages"=w156) -> ("Error Out"=w158:errorcluster)  [unwired: 5 in, 1 out]
            n48 = disable-structure shown="Disabled" {
              disable-tunnel: w158 -> [w181 w184]
              disable-tunnel: [w180 w184] -> w157
              disable-tunnel: w156 -> [w178 _]
              frame Disabled {
                n49 = call "XYZ Table Stage Module.vi"("Set/Get"=Set_Get_Controls."Set", "Action"=Motion_Translation_Module_Control."Home", "Error In"=w181, "Axis"=enum16{"X Axis", "Y Axis", "Z Axis"}."Z Axis", "Table Stages"=w178) -> ("Error Out"=w180:errorcluster)  [unwired: 5 in, 1 out]
              }
              frame Enabled {
              }
            }
          }
        }
      }
      frame "Init Vibratome" {
        n50 = call "System Parameters - FGV.vi"("Actions"=FGV_Actions."Get", "Error In"=w189) -> ("Error Out"=w187:errorcluster, "System Parameters [Out]"=w186:T16)  [unwired: 8 in]
        n51 = Unbundle By Name(w186) -> ("Manual Controls.Acquisition mode"=w185:T33)
        n52 = case shown="\"GPU FFT\", Default" w185 {
          tunnel: [w195 w201] -> w190
          tunnel: w187 -> [w195 w197]
          tunnel: w186 -> [_ w196]
          frame "Simulation" {
          }
          frame "GPU FFT", Default {
            n53 = Unbundle By Name(w196) -> ("Table Stages"=w199:T19, "Vibratome"=w198:T18)
            n54 = call "Slice Engine.vi"("Table Stages"=w199, "error in (no error)"=w197, "Vibratome"=w198, "Action"="Configure Vibratome HW") -> ("error out"=w201:errorcluster)  [unwired: 7 in]
          }
        }
      }
      frame "Generate Mosaic" {
        n55 = call "System Parameters - FGV.vi"("Actions"=FGV_Actions."Get", "Error In"=w205) -> ("Error Out"=w204:errorcluster, "System Parameters [Out]"=w203:T16)  [unwired: 8 in]
        n56 = Unbundle By Name(w203) -> ("Mosaic Paramter"=w213:T35)
        n57 = Unbundle By Name(w213) -> ("X Axis"=w217:T36, "Y Axis"=w216:T36, "Overlap Options"=w215:T37, "Scan Pattern"=w214:T38)
        n58 = call "Calculate X Y Step Size.vi"("Overlap Options"=w215, "Scan Pattern"=w214, "Error In"=w204, "Y Axis"=w216, "X Axis"=w217) -> ("Error Out"=w209:errorcluster, "Array"=w208:cluster{"X":dbl, "Y":dbl}[])  [unwired: 3 in, 2 out]
        n59 = Array Size(array=w208) -> (size(s)=w207:i32)
        n60 = call "Tile naming.vi"(7:Tile_naming_actions."Total tile num", "Error In"=w209, "Tile Num"=w207) -> ("Error Out"=w202:errorcluster)  [unwired: 5 in, 3 out]
      }
      frame "Go Image Home" {
        n61 = call "System Parameters - FGV.vi"("Actions"=FGV_Actions."Get", "Error In"=w222) -> ("Error Out"=w221:errorcluster, "System Parameters [Out]"=w220:T16)  [unwired: 8 in]
        n62 = Unbundle By Name(w220) -> ("Manual Controls.Acquisition mode"=w219:T33)
        n63 = case shown="\"GPU FFT\", Default" w219 {
          tunnel: [w229 w247] -> w224
          tunnel: w221 -> [w229 w236]
          tunnel: w220 -> [_ w235]
          frame "Simulation" {
          }
          frame "GPU FFT", Default {
            n64 = Unbundle By Name(w235) -> ("Mosaic Paramter.X Axis"=w257:T36, "Mosaic Paramter.Y Axis"=w256:T36)
            n65 = Unbundle By Name(w257) -> ("End [mm]"=w249:dbl)
            n66 = Unbundle By Name(w256) -> ("End [mm]"=w248:dbl)
            n67 = Unbundle By Name(w235) -> ("Table Stages"=w250:T19)
            n68 = Bundle By Name(cluster=w250, "X Stage.Position"=w249, "Y Stage.Position"=w248) -> (w237:T19)
            n69 = call "XYZ Table Stage Module.vi"("Set/Get"=Set_Get_Controls."Set", "Action"=Motion_Translation_Module_Control2."Velocity/Accel", "Error In"=w236, "Axis"=enum16{"X Axis", "Y Axis", "Z Axis"}."X Axis", "Table Stages"=w237) -> ("Error Out"=w246:errorcluster)  [unwired: 5 in, 1 out]
            n70 = call "XYZ Table Stage Module.vi"("Set/Get"=Set_Get_Controls."Set", "Action"=Motion_Translation_Module_Control2."Velocity/Accel", "Error In"=w246, "Axis"=enum16{"X Axis", "Y Axis", "Z Axis"}."Y Axis", "Table Stages"=w237) -> ("Error Out"=w241:errorcluster)  [unwired: 5 in, 1 out]
            n71 = call "XYZ Table Stage Module.vi"("Set/Get"=Set_Get_Controls."Set", "Action"=Motion_Translation_Module_Control2."Velocity/Accel", "Error In"=w241, "Axis"=enum16{"X Axis", "Y Axis", "Z Axis"}."Z Axis", "Table Stages"=w237) -> ("Error Out"=w238:errorcluster)  [unwired: 5 in, 1 out]
            n72 = call "XYZ Table Stage Module.vi"("Set/Get"=Set_Get_Controls."Set", "Action"=Motion_Translation_Module_Control2."Position", "Error In"=w238, "Axis"=enum16{"X Axis", "Y Axis", "Z Axis"}."X Axis", "Table Stages"=w237) -> ("Error Out"=w251:errorcluster)  [unwired: 5 in, 1 out]
            n73 = call "XYZ Table Stage Module.vi"("Set/Get"=Set_Get_Controls."Set", "Action"=Motion_Translation_Module_Control2."Position", "Error In"=w251, "Axis"=enum16{"X Axis", "Y Axis", "Z Axis"}."Y Axis", "Table Stages"=w237) -> ("Error Out"=w247:errorcluster)  [unwired: 5 in, 1 out]
          }
        }
      }
      frame "Go to Image Z" {
        n74 = Empty Array?(array=w260) -> (empty?=w261:bool)
        n75 = case shown="False" w261 {
          tunnel: [w268 w284] -> w265
          tunnel: w263 -> [w268 w280]
          tunnel: w260 -> [w269 w279]
          tunnel: [w269 w278] -> w262
          tunnel: w259 -> [_ w276]
          tunnel: [w267 w276] -> w258
          frame True {
            w267 = T1[] [enum."Finished"] items=["Init(ThorOCT Spatial)", "Init(ThorOCT Spectral)", "Init(GPU FFT)", "Init(Alazar FFT)", "Init Scan Head(ThorOCT Spectral)", "Init Scan Head(ThorOCT Spatial)", "Init Scan Head", "Init Table Stage", "Init Vibratome", "Generate Mosaic", "Generate Z Position", "Go to Image Z", "Go Image Home", "Go Mosaic", "Acquire Image(ThorOCT Spatial)", "Acquire Image(ThorOCT Spectral)", "Acquire Image(GPU FFT)", "Acquire Image(Alazar FFT)", "Go Vibratome", "Slice", "Finished(ThorOCT)", "Finished", "Init(Alazar Spectral)", "Go Vibratome3"]
          }
          frame False {
            n76 = flat-sequence {
              tunnel: w280 -> [w302]
              tunnel: [w296] -> w273
              tunnel: w277 -> [w295]
              frame #0 {
                # "update image plane"
                n77 = call "Scan engine status.vi"("Actions"=FGV_Actions."Get", "Error In"=w302) -> ("slice plane out"=w301:dbl, "XY Graph out"=w300:cluster{"X":dbl, "Y":dbl}[], "Current Position out"=w299:cluster{"X":dbl, "Y":dbl}, "Current state out"=w298:T1, "Error Out"=w297:errorcluster)  [unwired: 8 in, 1 out]
                n78 = call "Scan engine status.vi"("XY Graph in"=w300, "Actions"=FGV_Actions."Set", "Current Position in"=w299, "Current state in"=w298, "Error In"=w297, "image plane"=w295, "slice plane"=w301) -> ("Error Out"=w296:errorcluster)  [unwired: 3 in, 5 out]
              }
            }
            n79 = Delete From Array(array=w279, length=1, index=0) -> (deleted portion=w275:dbl[], array with subset deleted=w278:dbl[])
            n80 = Index Array(array=w275, index=0) -> (element=w277:dbl)
            n81 = call "System Parameters - FGV.vi"("Actions"=FGV_Actions."Get", "Error In"=w273) -> ("Error Out"=w272:errorcluster, "System Parameters [Out]"=w271:T16)  [unwired: 8 in]
            n82 = Unbundle By Name(w271) -> ("Manual Controls.Acquisition mode"=w270:T33)
            n83 = case shown="\"GPU FFT\", Default" w270 {
              tunnel: [w285 w292] -> w284
              tunnel: w277 -> [_ w289]
              tunnel: w271 -> [_ w288]
              tunnel: w272 -> [w285 w287]
              frame "Simulation" {
              }
              frame "GPU FFT", Default {
                n84 = Unbundle By Name(w288) -> ("Table Stages"=w291:T19)
                n85 = Bundle By Name(cluster=w291, "Z Stage.Position"=w289) -> (w290:T19)
                n86 = call "XYZ Table Stage Module.vi"("Set/Get"=Set_Get_Controls."Set", "Action"=Motion_Translation_Module_Control2."Position", "Error In"=w287, "Axis"=enum16{"X Axis", "Y Axis", "Z Axis"}."Z Axis", "Table Stages"=w290) -> ("Error Out"=w292:errorcluster)  [unwired: 5 in, 1 out]
              }
            }
          }
        }
      }
      frame "Acquire Image(Alazar FFT)" {
        n87 = call "FGV - Acquisition Status.vi"("Actions"=FGV_Actions."Get", "Error In"=w310) -> ("Error Out"=w307:errorcluster, "Quit status out"=w311:bool, "Scan Type [Out]"=w314:T15)  [unwired: 6 in, 1 out]
        n88 = call "System Parameters - FGV.vi"("Actions"=FGV_Actions."Get", "Error In"=w307) -> ("Error Out"=w306:errorcluster, "System Parameters [Out]"=w308:T16)  [unwired: 8 in]
        n89 = Unbundle By Name(w308) -> ("Manual Controls.Acquisition mode"=w305:T33)
        n90 = case shown="\"GPU FFT\", Default" w305 {
          tunnel: [w320 w323] -> w312
          tunnel: w306 -> [w320 w321]
          frame "Simulation" {
          }
          frame "GPU FFT", Default {
            n91 = call "Image Acquiring Module.vi"("Scan Status in"=scan_status."Start(Alazar FFT)" ("Scan Status in 2"), "Error in"=w321) -> ("Error Out"=w326:errorcluster)  [unwired: 9 in]
            n92 = call "AlazarEngine.vi"("error in (no error)"=w326, "Action"=Alazar_Engine_Actions."start acquire") -> ("error out"=w329:errorcluster)  [unwired: 15 in, 2 out]
            n93 = call "Galvo Module.vi"("Action"=T10."Start Galvo Task", "error in (no error)"=w329) -> ("error out"=w333:errorcluster)  [unwired: 8 in, 1 out]
            n94 = call "Image Acquiring Module.vi"("Scan Status in"=scan_status."Scan(Alazar FFT)", "Error in"=w333) -> ("Error Out"=w325:errorcluster)  [unwired: 9 in]
            n95 = call "Image Acquiring Module.vi"("Scan Status in"=scan_status."Complete Scan(PSOCT)" ("Scan Status in 2"), "Error in"=w325) -> ("Error Out"=w324:errorcluster)  [unwired: 9 in]
            n96 = call "Image Acquiring Module.vi"("Scan Status in"=scan_status."Finish Scan(PSOCT)", "Error in"=w324) -> ("Error Out"=w323:errorcluster)  [unwired: 9 in]
          }
        }
        n97 = case shown="False" w311 {
          tunnel: w316 -> [w334 w337]
          tunnel: w314 -> [_ w336]
          tunnel: [w334 w335] -> w313
          frame True {
          }
          frame False {
            n98 = case shown="\"Continuous Frame\"" w336 {
              tunnel: w337 -> [w338 w340]
              tunnel: [w338 w342] -> w335
              frame "Single Frame", Default {
              }
              frame "Continuous Frame" {
                w341 = T1[] [enum."Acquire Image(Alazar FFT)"] items=["Init(ThorOCT Spatial)", "Init(ThorOCT Spectral)", "Init(GPU FFT)", "Init(Alazar FFT)", "Init Scan Head(ThorOCT Spectral)", "Init Scan Head(ThorOCT Spatial)", "Init Scan Head", "Init Table Stage", "Init Vibratome", "Generate Mosaic", "Generate Z Position", "Go to Image Z", "Go Image Home", "Go Mosaic", "Acquire Image(ThorOCT Spatial)", "Acquire Image(ThorOCT Spectral)", "Acquire Image(GPU FFT)", "Acquire Image(Alazar FFT)", "Go Vibratome", "Slice", "Finished(ThorOCT)", "Finished", "Init(Alazar Spectral)", "Go Vibratome3"]
                n99 = Build Array (concatenate)(w341, w340) -> (w342:T1[])
                n100 = Wait (ms)(milliseconds to wait=u32 1000) -> ()  [unwired: 1 out]
              }
            }
          }
        }
      }
      frame "Acquire Image(GPU FFT)" {
        n101 = call "FGV - Acquisition Status.vi"("Actions"=FGV_Actions."Get", "Error In"=w353) -> ("Error Out"=w346:errorcluster, "Quit status out"=w351:bool, "Scan Type [Out]"=w352:T15)  [unwired: 6 in, 1 out]
        n102 = call "System Parameters - FGV.vi"("Actions"=FGV_Actions."Get", "Error In"=w346) -> ("Error Out"=w345:errorcluster, "System Parameters [Out]"=w347:T16)  [unwired: 8 in]
        n103 = Unbundle By Name(w347) -> ("Manual Controls.Acquisition mode"=w344:T33)
        n104 = case shown="\"GPU FFT\", Default" w344 {
          tunnel: [w366 w371] -> w359
          tunnel: w345 -> [w363 w370]
          frame "Simulation" {
            n105 = call "Image Acquiring Module.vi"("Scan Status in"=scan_status."Start(GPU FFT)" ("Scan Status in 2"), "Error in"=w363) -> ("Error Out"=w362:errorcluster)  [unwired: 9 in]
            n106 = call "Image Acquiring Module.vi"("Scan Status in"=scan_status."Scan(simulate)", "Error in"=w362) -> ("Error Out"=w366:errorcluster)  [unwired: 9 in]
          }
          frame "GPU FFT", Default {
            n107 = call "Image Acquiring Module.vi"("Scan Status in"=scan_status."Start(GPU FFT)" ("Scan Status in 2"), "Error in"=w370) -> ("Error Out"=w372:errorcluster)  [unwired: 9 in]
            n108 = call "AlazarEngine.vi"("error in (no error)"=w372, "Action"=Alazar_Engine_Actions."start acquire") -> ("error out"=w368:errorcluster)  [unwired: 15 in, 2 out]
            n109 = call "Galvo Module.vi"("Action"=T10."Start Galvo Task", "error in (no error)"=w368) -> ("error out"=w375:errorcluster)  [unwired: 8 in, 1 out]
            n110 = call "Image Acquiring Module.vi"("Scan Status in"=scan_status."Scan(GPU FFT)", "Error in"=w375) -> ("Error Out"=w371:errorcluster)  [unwired: 9 in]
          }
        }
        n111 = case shown="False" w351 {
          tunnel: w356 -> [w376 w379]
          tunnel: w352 -> [_ w378]
          tunnel: [w376 w377] -> w355
          frame True {
          }
          frame False {
            n112 = case shown="\"Single Frame\", Default" w378 {
              tunnel: w379 -> [w380 w382]
              tunnel: [w380 w384] -> w377
              frame "Single Frame", Default {
              }
              frame "Continuous Frame" {
                w383 = T1[] [enum."Acquire Image(GPU FFT)"] items=["Init(ThorOCT Spatial)", "Init(ThorOCT Spectral)", "Init(GPU FFT)", "Init(Alazar FFT)", "Init Scan Head(ThorOCT Spectral)", "Init Scan Head(ThorOCT Spatial)", "Init Scan Head", "Init Table Stage", "Init Vibratome", "Generate Mosaic", "Generate Z Position", "Go to Image Z", "Go Image Home", "Go Mosaic", "Acquire Image(ThorOCT Spatial)", "Acquire Image(ThorOCT Spectral)", "Acquire Image(GPU FFT)", "Acquire Image(Alazar FFT)", "Go Vibratome", "Slice", "Finished(ThorOCT)", "Finished", "Init(Alazar Spectral)", "Go Vibratome3"]
                n113 = Build Array (concatenate)(w383, w382) -> (w384:T1[])
                n114 = Wait (ms)(milliseconds to wait=u32 1100) -> ()  [unwired: 1 out]
              }
            }
          }
        }
        n115 = call "Image Acquiring Module.vi"("Scan Status in"=scan_status."Complete Scan(PSOCT)" ("Scan Status in 2"), "Error in"=w359) -> ("Error Out"=w350:errorcluster)  [unwired: 9 in]
        n116 = call "Image Acquiring Module.vi"("Scan Status in"=scan_status."Finish Scan(PSOCT)" ("Scan Status in 2"), "Error in"=w350) -> ("Error Out"=w343:errorcluster)  [unwired: 9 in]
      }
      frame "Go Mosaic" {
        n117 = Delete From Array(array=w387) -> (deleted portion=w389:cluster{"X":dbl, "Y":dbl}, array with subset deleted=w392:cluster{"X":dbl, "Y":dbl}[])  [unwired: 2 in]
        n118 = Empty Array?(array=w387) -> (empty?=w393:bool)
        n119 = case shown="False" w393 {
          tunnel: [w409 w476] -> w396
          tunnel: w392 -> [w409 w476]
          tunnel: [w412 w474] -> w394
          tunnel: [w399 w475] -> w395
          tunnel: w389 -> [w400 _]
          tunnel: w385 -> [w402 w475]
          tunnel: w386 -> [w405 w474]
          tunnel: w388 -> [w404 _]
          tunnel: w387 -> [w403 _]
          frame False {
            n120 = flat-sequence {
              tunnel: w400 -> [w437]
              tunnel: w404 -> [w446]
              tunnel: w402 -> [w444]
              tunnel: w403 -> [w430]
              tunnel: [w424] -> w401
              frame #0 {
                # "update XY stage position"
                n121 = call "Scan engine status.vi"("Actions"=FGV_Actions."Get", "Error In"=w444) -> ("slice plane out"=w434:dbl, "image plane out"=w433:dbl, "Error Out"=w443:errorcluster)  [unwired: 8 in, 3 out]
                n122 = call "Scan engine status.vi"("XY Graph in"=w430, "Actions"=FGV_Actions."Set", "Current Position in"=w437, "Current state in"=w446, "Error In"=w443, "image plane"=w433, "slice plane"=w434) -> ("Error Out"=w442:errorcluster)  [unwired: 3 in, 5 out]
                n123 = Unbundle By Name(w437) -> ("X"=w436:dbl, "Y"=w435:dbl)
                n124 = call "file log variable.vi"("X stage position"=w436, "error in"=w442, "Item"=file_variable_action."X stage") -> ("error out"=w441:errorcluster)  [unwired: 15 in, 1 out]
                n125 = call "file log variable.vi"("Y stage position"=w435, "error in"=w441, "Item"=file_variable_action."Y stage") -> ("error out"=w440:errorcluster)  [unwired: 15 in, 1 out]
                n126 = call "file log variable.vi"("slice plane"=w434, "error in"=w440, "Item"=file_variable_action."Slice plane") -> ("error out"=w439:errorcluster)  [unwired: 15 in, 1 out]
                n127 = Get Date/Time In Seconds() -> (seconds since 1Jan1904=w432:timestamp)
                n128 = call "file log variable.vi"("error in"=w439, "image plane"=w433, "Item"=file_variable_action."Image plane") -> ("error out"=w438:errorcluster)  [unwired: 15 in, 1 out]
                n129 = Format Date/Time String(seconds (now)=w432) -> (date/time string=w431:string)  [unwired: 2 in]
                n130 = call "file log variable.vi"("error in"=w438, "time"=w431, "Item"=file_variable_action."time") -> ("error out"=w424:errorcluster)  [unwired: 15 in, 1 out]
              }
            }
            n131 = call "System Parameters - FGV.vi"("Actions"=FGV_Actions."Get", "Error In"=w401) -> ("Error Out"=w407:errorcluster, "System Parameters [Out]"=w406:T16)  [unwired: 8 in]
            n132 = Unbundle By Name(w406) -> ("Table Stages"=w410:T19, "Manual Controls.Acquisition mode"=w398:T33)
            n133 = case shown="\"GPU FFT\", Default" w398 {
              tunnel: w410 -> [_ w459]
              tunnel: w400 -> [_ w453]
              tunnel: [w448 w452] -> w397
              tunnel: w407 -> [w448 w451]
              frame "Simulation" {
              }
              frame "GPU FFT", Default {
                n134 = Unbundle By Name(w453) -> ("X"=w458:dbl, "Y"=w457:dbl)
                n135 = Bundle By Name(cluster=w459, "X Stage.Position"=w458, "Y Stage.Position"=w457) -> (w456:T19)
                n136 = call "XYZ Table Stage Module.vi"("Set/Get"=Set_Get_Controls."Set", "Action"=Motion_Translation_Module_Control2."Position", "Error In"=w451, "Axis"=enum16{"X Axis", "Y Axis", "Z Axis"}."X Axis", "Table Stages"=w456) -> ("Error Out"=w454:errorcluster)  [unwired: 5 in, 1 out]
                n137 = call "XYZ Table Stage Module.vi"("Set/Get"=Set_Get_Controls."Set", "Action"=Motion_Translation_Module_Control2."Position", "Error In"=w451, "Axis"=enum16{"X Axis", "Y Axis", "Z Axis"}."Y Axis", "Table Stages"=w456) -> ("Error Out"=w455:errorcluster)  [unwired: 5 in, 1 out]
                n138 = Merge Errors(w454, w455) -> (w452:errorcluster)
              }
            }
            n139 = case shown="\"Alazar Spectral\"" w398 {
              tunnel: [w464 w465 w466 w470 w471 w472] -> w411
              frame "Alazar FFT", Default {
                w464 = T1[] [enum."Acquire Image(Alazar FFT)", enum."Go Mosaic"] items=["Init(ThorOCT Spatial)", "Init(ThorOCT Spectral)", "Init(GPU FFT)", "Init(Alazar FFT)", "Init Scan Head(ThorOCT Spectral)", "Init Scan Head(ThorOCT Spatial)", "Init Scan Head", "Init Table Stage", "Init Vibratome", "Generate Mosaic", "Generate Z Position", "Go to Image Z", "Go Image Home", "Go Mosaic", "Acquire Image(ThorOCT Spatial)", "Acquire Image(ThorOCT Spectral)", "Acquire Image(GPU FFT)", "Acquire Image(Alazar FFT)", "Go Vibratome", "Slice", "Finished(ThorOCT)", "Finished", "Init(Alazar Spectral)", "Go Vibratome3"]
              }
              frame "Alazar B line" {
                w465 = T1[] [enum."Acquire Image(Alazar FFT)", enum."Go Mosaic"] items=["Init(ThorOCT Spatial)", "Init(ThorOCT Spectral)", "Init(GPU FFT)", "Init(Alazar FFT)", "Init Scan Head(ThorOCT Spectral)", "Init Scan Head(ThorOCT Spatial)", "Init Scan Head", "Init Table Stage", "Init Vibratome", "Generate Mosaic", "Generate Z Position", "Go to Image Z", "Go Image Home", "Go Mosaic", "Acquire Image(ThorOCT Spatial)", "Acquire Image(ThorOCT Spectral)", "Acquire Image(GPU FFT)", "Acquire Image(Alazar FFT)", "Go Vibratome", "Slice", "Finished(ThorOCT)", "Finished", "Init(Alazar Spectral)", "Go Vibratome3"]
              }
              frame "Alazar Spectral" {
                w466 = T1[] [enum."Acquire Image(GPU FFT)", enum."Go Mosaic"] items=["Init(ThorOCT Spatial)", "Init(ThorOCT Spectral)", "Init(GPU FFT)", "Init(Alazar FFT)", "Init Scan Head(ThorOCT Spectral)", "Init Scan Head(ThorOCT Spatial)", "Init Scan Head", "Init Table Stage", "Init Vibratome", "Generate Mosaic", "Generate Z Position", "Go to Image Z", "Go Image Home", "Go Mosaic", "Acquire Image(ThorOCT Spatial)", "Acquire Image(ThorOCT Spectral)", "Acquire Image(GPU FFT)", "Acquire Image(Alazar FFT)", "Go Vibratome", "Slice", "Finished(ThorOCT)", "Finished", "Init(Alazar Spectral)", "Go Vibratome3"]
                n140 = disable-structure shown="Enabled" {
                  frame Disabled {
                    n141 = while {
                      stop <- w468 stop-if-true
                      n142 = call "Process status.vi"("Actions"=FGV_Actions."Get") -> ("Status Out"=w468:bool)  [unwired: 9 in, 1 out]
                      n143 = Wait (ms)(milliseconds to wait=u32 500) -> ()  [unwired: 1 out]
                    }
                  }
                  frame Enabled {
                  }
                }
              }
              frame "GPU FFT" {
                w470 = T1[] [enum."Acquire Image(GPU FFT)", enum."Go Mosaic"] items=["Init(ThorOCT Spatial)", "Init(ThorOCT Spectral)", "Init(GPU FFT)", "Init(Alazar FFT)", "Init Scan Head(ThorOCT Spectral)", "Init Scan Head(ThorOCT Spatial)", "Init Scan Head", "Init Table Stage", "Init Vibratome", "Generate Mosaic", "Generate Z Position", "Go to Image Z", "Go Image Home", "Go Mosaic", "Acquire Image(ThorOCT Spatial)", "Acquire Image(ThorOCT Spectral)", "Acquire Image(GPU FFT)", "Acquire Image(Alazar FFT)", "Go Vibratome", "Slice", "Finished(ThorOCT)", "Finished", "Init(Alazar Spectral)", "Go Vibratome3"]
              }
              frame "Save all" {
                w471 = T1[] [enum."Acquire Image(GPU FFT)", enum."Go Mosaic"] items=["Init(ThorOCT Spatial)", "Init(ThorOCT Spectral)", "Init(GPU FFT)", "Init(Alazar FFT)", "Init Scan Head(ThorOCT Spectral)", "Init Scan Head(ThorOCT Spatial)", "Init Scan Head", "Init Table Stage", "Init Vibratome", "Generate Mosaic", "Generate Z Position", "Go to Image Z", "Go Image Home", "Go Mosaic", "Acquire Image(ThorOCT Spatial)", "Acquire Image(ThorOCT Spectral)", "Acquire Image(GPU FFT)", "Acquire Image(Alazar FFT)", "Go Vibratome", "Slice", "Finished(ThorOCT)", "Finished", "Init(Alazar Spectral)", "Go Vibratome3"]
              }
              frame "Simulation" {
                w472 = T1[] [enum."Acquire Image(GPU FFT)", enum."Go Mosaic"] items=["Init(ThorOCT Spatial)", "Init(ThorOCT Spectral)", "Init(GPU FFT)", "Init(Alazar FFT)", "Init Scan Head(ThorOCT Spectral)", "Init Scan Head(ThorOCT Spatial)", "Init Scan Head", "Init Table Stage", "Init Vibratome", "Generate Mosaic", "Generate Z Position", "Go to Image Z", "Go Image Home", "Go Mosaic", "Acquire Image(ThorOCT Spatial)", "Acquire Image(ThorOCT Spectral)", "Acquire Image(GPU FFT)", "Acquire Image(Alazar FFT)", "Go Vibratome", "Slice", "Finished(ThorOCT)", "Finished", "Init(Alazar Spectral)", "Go Vibratome3"]
              }
            }
            n144 = Build Array (concatenate)(w411, w405) -> (w412:T1[])
            n145 = while {
              tunnel: w397 -> [w416]
              tunnel: [w414] -> w399
              stop <- w417 stop-if-true
              n146 = call "Pause.vi"("action"=Pause_action."get", "error in"=w416) -> ("error out"=w415:errorcluster, "Pause?"=w418:bool)  [unwired: 8 in]
              n147 = Wait (ms)(milliseconds to wait=u32 200) -> ()  [unwired: 1 out]
              n148 = case shown="False" w418 {
                tunnel: [TRUE FALSE] -> w417
                tunnel: w415 -> [w420 w422]
                tunnel: [w420 w422] -> w414
                frame False {
                }
                frame True {
                }
              }
            }
          }
          frame True {
            n149 = Wait (ms)(milliseconds to wait=u32 5000) -> ()  [unwired: 1 out]
          }
        }
      }
      frame "Go Vibratome" {
        n150 = Empty Array?(array=w478) -> (empty?=w482:bool)
        n151 = Or(x=w477, y=w482) -> (x .or. y?=w481:bool)
        n152 = case shown="False" w481 {
          tunnel: w486 -> [w502 w712]
          tunnel: [w509 w712] -> w484
          tunnel: [w506 w711] -> w485
          tunnel: w483 -> [w496 w711]
          tunnel: [w488 _] -> w480
          tunnel: w478 -> [w508 _]
          frame False {
            w500 = T1[] [enum."Go Vibratome"] items=["Init(ThorOCT Spatial)", "Init(ThorOCT Spectral)", "Init(GPU FFT)", "Init(Alazar FFT)", "Init Scan Head(ThorOCT Spectral)", "Init Scan Head(ThorOCT Spatial)", "Init Scan Head", "Init Table Stage", "Init Vibratome", "Generate Mosaic", "Generate Z Position", "Go to Image Z", "Go Image Home", "Go Mosaic", "Acquire Image(ThorOCT Spatial)", "Acquire Image(ThorOCT Spectral)", "Acquire Image(GPU FFT)", "Acquire Image(Alazar FFT)", "Go Vibratome", "Slice", "Finished(ThorOCT)", "Finished", "Init(Alazar Spectral)", "Go Vibratome3"] ("array")
            w503 = T1[] [] items=["Init(ThorOCT Spatial)", "Init(ThorOCT Spectral)", "Init(GPU FFT)", "Init(Alazar FFT)", "Init Scan Head(ThorOCT Spectral)", "Init Scan Head(ThorOCT Spatial)", "Init Scan Head", "Init Table Stage", "Init Vibratome", "Generate Mosaic", "Generate Z Position", "Go to Image Z", "Go Image Home", "Go Mosaic", "Acquire Image(ThorOCT Spatial)", "Acquire Image(ThorOCT Spectral)", "Acquire Image(GPU FFT)", "Acquire Image(Alazar FFT)", "Go Vibratome", "Slice", "Finished(ThorOCT)", "Finished", "Init(Alazar Spectral)", "Go Vibratome3"]
            n153 = flat-sequence {
              tunnel: [w710] -> w488
              tunnel: w508 -> [w709]
              tunnel: [w701] -> w507
              frame #0 {
                n154 = Delete From Array(array=w709, length=1, index=0) -> (deleted portion=w706:dbl[], array with subset deleted=w710:dbl[])
                n155 = Index Array(array=w706, index=0) -> (element=w701:dbl)
                n156 = call "Scan engine status.vi"("Actions"=FGV_Actions."Get") -> ("image plane out"=w700:dbl, "XY Graph out"=w699:cluster{"X":dbl, "Y":dbl}[], "Current Position out"=w698:cluster{"X":dbl, "Y":dbl}, "Current state out"=w697:T1, "Error Out"=w702:errorcluster)  [unwired: 9 in, 1 out]
                n157 = call "Scan engine status.vi"("XY Graph in"=w699, "Actions"=FGV_Actions."Set", "Current Position in"=w698, "Current state in"=w697, "Error In"=w702, "image plane"=w700, "slice plane"=w701) -> ()  [unwired: 3 in, 6 out]
              }
            }
            n158 = call "System Parameters - FGV.vi"("Actions"=FGV_Actions."Get", "Error In"=w496) -> ("Error Out"=w495:errorcluster, "System Parameters [Out]"=w498:T16)  [unwired: 8 in]
            n159 = Unbundle By Name(w498) -> ("Table Stages"=w505:T19, "Vibratome"=w494:T18, "Manual Controls.Z0"=w497:dbl, "Manual Controls.Acquisition mode"=w491:T33, "Vibratome Axis.30um?"=w490:bool, "Manual Controls.blocker position"=w489:enum16{"every two slices", "Nat slices", "None"})
            n160 = case shown="\"GPU FFT\", Default" w491 {
              tunnel: w507 -> [_ w527]
              tunnel: [w510 w526] -> w506
              tunnel: w505 -> [_ w525]
              tunnel: w497 -> [_ w524]
              tunnel: w495 -> [w510 w515]
              tunnel: w494 -> [_ w523]
              tunnel: w490 -> [_ w514]
              tunnel: w489 -> [_ w512]
              tunnel: w488 -> [_ w511]
              frame "Simulation" {
              }
              frame "GPU FFT", Default {
                w518 = 2  # slice# for Nat
                w520 = 6  # #slices per cycle
                n161 = call "Tile naming.vi"(7:Tile_naming_actions."Export", "Error In"=w515) -> ("Error Out"=w516:errorcluster, "slice"=w521:i32)  [unwired: 6 in, 2 out]
                n162 = Quotient & Remainder(x=w521, y=w520) -> (x-y*floor(x/y)=w519:i32)  [unwired: 1 out]
                n163 = Equal?(x=w518, y=w519) -> (x = y?=w517:bool)
                n164 = And(x=w514, y=w517) -> (x .and. y?=w513:bool)
                n165 = case shown="False" w513 {
                  tunnel: w527 -> [w543 w612]
                  tunnel: [w542 w611] -> w526
                  tunnel: w525 -> [w541 w610]
                  tunnel: w524 -> [w539 w605]
                  tunnel: w516 -> [w538 w606]
                  tunnel: w523 -> [w536 w609]
                  tunnel: w512 -> [w533 w603]
                  tunnel: w511 -> [w532 _]
                  frame False {
                    n166 = Bundle By Name(cluster=w541, "Z Stage.Position"=w539) -> (w540:T19)
                    n167 = flat-sequence {
                      tunnel: [w600] -> w550
                      tunnel: w538 -> [w599]
                      tunnel: w540 -> [w598]
                      frame #0 {
                        # "Go to Z0"
                        n168 = call "XYZ Table Stage Module.vi"("Set/Get"=Set_Get_Controls."Set", "Action"=Motion_Translation_Module_Control2."Position", "Error In"=w599, "Axis"=enum16{"X Axis", "Y Axis", "Z Axis"}."Z Axis", "Table Stages"=w598) -> ("Error Out"=w600:errorcluster)  [unwired: 5 in, 1 out]
                      }
                    }
                    n169 = Array Size(array=w532) -> (size(s)=w531:i32)
                    n170 = call "Slice Engine.vi"("Table Stages"=w541, "error in (no error)"=w550, "Vibratome"=w536, "Action"="Move Stage (XY)") -> ("error out"=w548:errorcluster)  [unwired: 7 in]
                    n171 = Quotient & Remainder(x=w531, y=2) -> (x-y*floor(x/y)=w529:i32)  [unwired: 1 out]
                    n172 = flat-sequence {
                      tunnel: w548 -> [w588]
                      tunnel: [w587] -> w547
                      tunnel: w544 -> [w586]
                      frame #0 {
                        # "Go to next cut height"
                        n173 = call "XYZ Table Stage Module.vi"("Set/Get"=Set_Get_Controls."Set", "Action"=Motion_Translation_Module_Control2."Position", "Error In"=w588, "Axis"=enum16{"X Axis", "Y Axis", "Z Axis"}."Z Axis", "Table Stages"=w586) -> ("Error Out"=w587:errorcluster)  [unwired: 5 in, 1 out]
                      }
                    }
                    n174 = Bundle By Name(cluster=w541, "Z Stage.Position"=w543) -> (w544:T19)
                    n175 = call "Slice Engine.vi"("Table Stages"=w541, "error in (no error)"=w547, "Vibratome"=w536, "Action"="Set Slice Speed") -> ("error out"=w534:errorcluster)  [unwired: 7 in]
                    n176 = case shown="\"every two slices\"" w533 {
                      tunnel: w529 -> [_ w556]
                      tunnel: w534 -> [w551 w553]
                      tunnel: [w551 w552] -> w535
                      frame "None", Default {
                      }
                      frame "every two slices" {
                        n177 = Equal?(x=w556, y=1) -> (x = y?=w554:bool)
                        n178 = case shown="True" w554 {
                          tunnel: w553 -> [w557 w571]
                          tunnel: [w557 w569] -> w552
                          frame False {
                          }
                          frame True {
                            n179 = call "Pause.vi"("action"=Pause_action."set", "error in"=w571, "Pause!"=TRUE) -> ("error out"=w570:errorcluster)  [unwired: 7 in, 1 out]
                            n180 = call "System Parameters - FGV.vi"("Actions"=FGV_Actions."Get", "Error In"=w570) -> ("Error Out"=w569:errorcluster, "System Parameters [Out]"=w567:T16)  [unwired: 8 in]
                            n181 = Unbundle By Name(w567) -> ("Manual Controls.Outgoing Mail Server (SMTP)"=w560:string, "Manual Controls.Email"=w564:string, "Manual Controls.Password"=w563:string, "Manual Controls.Carrier 1"=w566:enum16{"T-Mobile", "AT&T", "Verizon", "Sprint"}, "Manual Controls.phone number 1"=w565:string, "Manual Controls.Subject"=w562:string, "Manual Controls.Message"=w561:string, "Manual Controls.phone number 2"=w559:string, "Manual Controls.Carrier 2"=w558:enum16{"T-Mobile", "AT&T", "Verizon", "Sprint"})
                            n182 = call "Send Text Using SMTP API 2013 NIVerified.vi"("phone number 2"=w559, "Carrier 2"=w558, "Body"=w561, "Carrier 1"=w566, "Subject"=w562, "phone number 1"=w565, "Outgoing Mail Server (SMTP)"=w560, "Password"=w563, "Email"=w564) -> ()  [unwired: 3 in]
                          }
                        }
                      }
                    }
                    n183 = while {
                      tunnel: w535 -> [w577]
                      tunnel: [w575] -> w528
                      stop <- w578 stop-if-true
                      n184 = call "Pause.vi"("action"=Pause_action."get", "error in"=w577) -> ("error out"=w576:errorcluster, "Pause?"=w579:bool)  [unwired: 8 in]
                      n185 = Wait (ms)(milliseconds to wait=u32 200) -> ()  [unwired: 1 out]
                      n186 = case shown="False" w579 {
                        tunnel: [TRUE FALSE] -> w578
                        tunnel: w576 -> [w581 w583]
                        tunnel: [w581 w583] -> w575
                        frame False {
                        }
                        frame True {
                        }
                      }
                    }
                    n187 = call "Slice Engine.vi"("Table Stages"=w541, "error in (no error)"=w528, "Vibratome"=w536, "Action"="Slice") -> ("error out"=w545:errorcluster)  [unwired: 7 in]
                    n188 = flat-sequence {
                      tunnel: w545 -> [w594]
                      tunnel: [w593] -> w542
                      tunnel: w540 -> [w592]
                      frame #0 {
                        # "Go to Z0"
                        n189 = call "XYZ Table Stage Module.vi"("Set/Get"=Set_Get_Controls."Set", "Action"=Motion_Translation_Module_Control2."Position", "Error In"=w594, "Axis"=enum16{"X Axis", "Y Axis", "Z Axis"}."Z Axis", "Table Stages"=w592) -> ("Error Out"=w593:errorcluster)  [unwired: 5 in, 1 out]
                      }
                    }
                  }
                  frame True {
                    n190 = Bundle By Name(cluster=w610, "Z Stage.Position"=w605) -> (w607:T19)
                    n191 = flat-sequence {
                      tunnel: [w616] -> w604
                      tunnel: w606 -> [w615]
                      tunnel: w607 -> [w614]
                      frame #0 {
                        # "Go to Z0"
                        n192 = call "XYZ Table Stage Module.vi"("Set/Get"=Set_Get_Controls."Set", "Action"=Motion_Translation_Module_Control2."Position", "Error In"=w615, "Axis"=enum16{"X Axis", "Y Axis", "Z Axis"}."Z Axis", "Table Stages"=w614) -> ("Error Out"=w616:errorcluster)  [unwired: 5 in, 1 out]
                      }
                    }
                    n193 = for {
                      N: 5 -> [_]
                      tunnel: w612 -> [w636]
                      tunnel: w610 -> [w625]
                      tunnel: w609 -> [w640]
                      shift-right: [w626] -> w611
                      shift-left: w604 -> [w624]
                      tunnel: w603 -> [w623]
                      i -> [w622]
                      n194 = Subtract(x=w636, y=0.12) -> (x-y=w633:dbl)
                      n195 = Multiply(x=w622, y=0.03) -> (x*y=w637:dbl)
                      n196 = Add(x=w633, y=w637) -> (x+y=w635:dbl)
                      n197 = call "Slice Engine.vi"("Table Stages"=w625, "error in (no error)"=w624, "Vibratome"=w640, "Action"="Move Stage (XY)") -> ("error out"=w646:errorcluster)  [unwired: 7 in]
                      n198 = flat-sequence {
                        tunnel: w646 -> [w685]
                        tunnel: [w684] -> w645
                        tunnel: w642 -> [w683]
                        frame #0 {
                          # "Go to next cut height"
                          n199 = call "XYZ Table Stage Module.vi"("Set/Get"=Set_Get_Controls."Set", "Action"=Motion_Translation_Module_Control2."Position", "Error In"=w685, "Axis"=enum16{"X Axis", "Y Axis", "Z Axis"}."Z Axis", "Table Stages"=w683) -> ("Error Out"=w684:errorcluster)  [unwired: 5 in, 1 out]
                        }
                      }
                      n200 = Bundle By Name(cluster=w625, "Z Stage.Position"=w635) -> (w642:T19)
                      n201 = call "Slice Engine.vi"("Table Stages"=w625, "error in (no error)"=w645, "Vibratome"=w640, "Action"="Set Slice Speed") -> ("error out"=w621:errorcluster)  [unwired: 7 in]
                      n202 = case shown="\"Nat slices\"" w623 {
                        tunnel: w622 -> [_ w653]
                        tunnel: w621 -> [w648 w651]
                        tunnel: [w648 w649] -> w620
                        frame "every two slices", Default {
                        }
                        frame "Nat slices" {
                          n203 = Equal?(x=w653, y=2) -> (x = y?=w650:bool)
                          n204 = case shown="True" w650 {
                            tunnel: w651 -> [w654 w668]
                            tunnel: [w654 w666] -> w649
                            frame False {
                            }
                            frame True {
                              n205 = call "Pause.vi"("action"=Pause_action."set", "error in"=w668, "Pause!"=TRUE) -> ("error out"=w667:errorcluster)  [unwired: 7 in, 1 out]
                              n206 = call "System Parameters - FGV.vi"("Actions"=FGV_Actions."Get", "Error In"=w667) -> ("Error Out"=w666:errorcluster, "System Parameters [Out]"=w664:T16)  [unwired: 8 in]
                              n207 = Unbundle By Name(w664) -> ("Manual Controls.Outgoing Mail Server (SMTP)"=w657:string, "Manual Controls.Email"=w661:string, "Manual Controls.Password"=w660:string, "Manual Controls.Carrier 1"=w663:enum16{"T-Mobile", "AT&T", "Verizon", "Sprint"}, "Manual Controls.phone number 1"=w662:string, "Manual Controls.Subject"=w659:string, "Manual Controls.Message"=w658:string, "Manual Controls.phone number 2"=w655:string, "Manual Controls.Carrier 2"=w656:enum16{"T-Mobile", "AT&T", "Verizon", "Sprint"})
                              n208 = call "Send Text Using SMTP API 2013 NIVerified.vi"("phone number 2"=w655, "Carrier 2"=w656, "Body"=w658, "Carrier 1"=w663, "Subject"=w659, "phone number 1"=w662, "Outgoing Mail Server (SMTP)"=w657, "Password"=w660, "Email"=w661) -> ()  [unwired: 3 in]
                            }
                          }
                        }
                      }
                      n209 = while {
                        tunnel: w620 -> [w674]
                        tunnel: [w672] -> w619
                        stop <- w675 stop-if-true
                        n210 = call "Pause.vi"("action"=Pause_action."get", "error in"=w674) -> ("error out"=w673:errorcluster, "Pause?"=w676:bool)  [unwired: 8 in]
                        n211 = Wait (ms)(milliseconds to wait=u32 200) -> ()  [unwired: 1 out]
                        n212 = case shown="False" w676 {
                          tunnel: [TRUE FALSE] -> w675
                          tunnel: w673 -> [w678 w680]
                          tunnel: [w678 w680] -> w672
                          frame False {
                          }
                          frame True {
                          }
                        }
                      }
                      n213 = Subtract(x=w633, y=0.1) -> (x-y=w632:dbl)
                      n214 = Bundle By Name(cluster=w625, "Z Stage.Position"=w632) -> (w631:T19)
                      n215 = call "Slice Engine.vi"("Table Stages"=w625, "error in (no error)"=w619, "Vibratome"=w640, "Action"="Slice") -> ("error out"=w643:errorcluster)  [unwired: 7 in]
                      n216 = flat-sequence {
                        tunnel: w643 -> [w691]
                        tunnel: [w690] -> w627
                        tunnel: w631 -> [w689]
                        frame #0 {
                          # "Go to Z0"
                          n217 = call "XYZ Table Stage Module.vi"("Set/Get"=Set_Get_Controls."Set", "Action"=Motion_Translation_Module_Control2."Position", "Error In"=w691, "Axis"=enum16{"X Axis", "Y Axis", "Z Axis"}."Z Axis", "Table Stages"=w689) -> ("Error Out"=w690:errorcluster)  [unwired: 5 in, 1 out]
                        }
                      }
                      n218 = call "XYZ Table Stage Module.vi"("Set/Get"=Set_Get_Controls."Set", "Action"=Motion_Translation_Module_Control2."Velocity/Accel", "Error In"=w627, "Axis"=enum16{"X Axis", "Y Axis", "Z Axis"}."X Axis", "Table Stages"=w625) -> ("Error Out"=w626:errorcluster)  [unwired: 5 in, 1 out]
                    }
                  }
                }
              }
            }
            n219 = call "System Parameters - FGV.vi"("Actions"=FGV_Actions."Get") -> ("System Parameters [Out]"=w492:T16)  [unwired: 9 in, 1 out]
            n220 = Unbundle By Name(w492) -> ("Vibratome Axis.#images"=w504:u16)
            n221 = for {
              N: w504 -> [_]
              shift-right: [w695] -> w501
              shift-left: w503 -> [w694]
              w696 = T1[] [enum."Generate Mosaic", enum."Go Image Home", enum."Go to Image Z", enum."Go Mosaic", enum."Init Scan Head"] items=["Init(ThorOCT Spatial)", "Init(ThorOCT Spectral)", "Init(GPU FFT)", "Init(Alazar FFT)", "Init Scan Head(ThorOCT Spectral)", "Init Scan Head(ThorOCT Spatial)", "Init Scan Head", "Init Table Stage", "Init Vibratome", "Generate Mosaic", "Generate Z Position", "Go to Image Z", "Go Image Home", "Go Mosaic", "Acquire Image(ThorOCT Spatial)", "Acquire Image(ThorOCT Spectral)", "Acquire Image(GPU FFT)", "Acquire Image(Alazar FFT)", "Go Vibratome", "Slice", "Finished(ThorOCT)", "Finished", "Init(Alazar Spectral)", "Go Vibratome3"]
              n222 = Build Array (concatenate)(w694, w696) -> (w695:T1[])
            }
            n223 = Build Array (concatenate)(w501, w500, w502) -> (w509:T1[])
          }
          frame True {
          }
        }
      }
      frame "Go Vibratome3" {
        n224 = Empty Array?(array=w714) -> (empty?=w718:bool)
        n225 = Or(x=w713, y=w718) -> (x .or. y?=w717:bool)
        n226 = case shown="False" w717 {
          tunnel: w722 -> [w738 w1083]
          tunnel: [w745 w1083] -> w720
          tunnel: [w742 w1082] -> w721
          tunnel: w719 -> [w732 w1082]
          tunnel: [w725 _] -> w716
          tunnel: w714 -> [w744 _]
          frame False {
            w736 = T1[] [enum."Go Vibratome3"] items=["Init(ThorOCT Spatial)", "Init(ThorOCT Spectral)", "Init(GPU FFT)", "Init(Alazar FFT)", "Init Scan Head(ThorOCT Spectral)", "Init Scan Head(ThorOCT Spatial)", "Init Scan Head", "Init Table Stage", "Init Vibratome", "Generate Mosaic", "Generate Z Position", "Go to Image Z", "Go Image Home", "Go Mosaic", "Acquire Image(ThorOCT Spatial)", "Acquire Image(ThorOCT Spectral)", "Acquire Image(GPU FFT)", "Acquire Image(Alazar FFT)", "Go Vibratome", "Slice", "Finished(ThorOCT)", "Finished", "Init(Alazar Spectral)", "Go Vibratome3"] ("array")
            w739 = T1[] [] items=["Init(ThorOCT Spatial)", "Init(ThorOCT Spectral)", "Init(GPU FFT)", "Init(Alazar FFT)", "Init Scan Head(ThorOCT Spectral)", "Init Scan Head(ThorOCT Spatial)", "Init Scan Head", "Init Table Stage", "Init Vibratome", "Generate Mosaic", "Generate Z Position", "Go to Image Z", "Go Image Home", "Go Mosaic", "Acquire Image(ThorOCT Spatial)", "Acquire Image(ThorOCT Spectral)", "Acquire Image(GPU FFT)", "Acquire Image(Alazar FFT)", "Go Vibratome", "Slice", "Finished(ThorOCT)", "Finished", "Init(Alazar Spectral)", "Go Vibratome3"]
            n227 = call "System Parameters - FGV.vi"("Actions"=FGV_Actions."Get", "Error In"=w732) -> ("Error Out"=w731:errorcluster, "System Parameters [Out]"=w734:T16)  [unwired: 8 in]
            n228 = Unbundle By Name(w734) -> ("Table Stages"=w741:T19, "Vibratome"=w730:T18, "Manual Controls.Z0"=w733:dbl, "Manual Controls.Acquisition mode"=w727:T33, "Vibratome Axis.30um?"=w726:bool, "Manual Controls.blocker position"=w724:enum16{"every two slices", "Nat slices", "None"})
            n229 = flat-sequence {
              tunnel: [w1081] -> w725
              tunnel: w744 -> [w1080]
              tunnel: [w1072] -> w743
              frame #0 {
                n230 = Delete From Array(array=w1080, length=1, index=0) -> (deleted portion=w1077:dbl[], array with subset deleted=w1081:dbl[])
                n231 = Index Array(array=w1077, index=0) -> (element=w1072:dbl)
                n232 = call "Scan engine status.vi"("Actions"=FGV_Actions."Get") -> ("image plane out"=w1071:dbl, "XY Graph out"=w1070:cluster{"X":dbl, "Y":dbl}[], "Current Position out"=w1069:cluster{"X":dbl, "Y":dbl}, "Current state out"=w1068:T1, "Error Out"=w1073:errorcluster)  [unwired: 9 in, 1 out]
                n233 = call "Scan engine status.vi"("XY Graph in"=w1070, "Actions"=FGV_Actions."Set", "Current Position in"=w1069, "Current state in"=w1068, "Error In"=w1073, "image plane"=w1071, "slice plane"=w1072) -> ()  [unwired: 3 in, 6 out]
              }
            }
            n234 = case shown="\"GPU FFT\", Default" w727 {
              tunnel: w743 -> [_ w763]
              tunnel: [w746 w762] -> w742
              tunnel: w741 -> [_ w759]
              tunnel: w733 -> [_ w760]
              tunnel: w731 -> [w746 w757]
              tunnel: w730 -> [_ w761]
              tunnel: [_ w759] -> _
              tunnel: [_ w761] -> _
              tunnel: w726 -> [_ w749]
              tunnel: w725 -> [_ w748]
              tunnel: w724 -> [_ w747]
              frame "Simulation" {
              }
              frame "GPU FFT", Default {
                w752 = 2  # slice# for Nat
                w754 = 6  # #slices per cycle
                n235 = call "Tile naming.vi"(7:Tile_naming_actions."Export", "Error In"=w757) -> ("Error Out"=w756:errorcluster, "slice"=w755:i32)  [unwired: 6 in, 2 out]
                n236 = Quotient & Remainder(x=w755, y=w754) -> (x-y*floor(x/y)=w753:i32)  [unwired: 1 out]
                n237 = Equal?(x=w752, y=w753) -> (x = y?=w751:bool)
                n238 = And(x=w749, y=w751) -> (x .and. y?=w750:bool)
                n239 = case shown="False" w750 {
                  tunnel: w763 -> [w796 w916]
                  tunnel: [w795 w915] -> w762
                  tunnel: w756 -> [w794 w910]
                  tunnel: w761 -> [w772 w912]
                  tunnel: w760 -> [w782 w909]
                  tunnel: w759 -> [w780 w913]
                  tunnel: w748 -> [w768 _]
                  tunnel: w747 -> [w764 w907]
                  frame False {
                    n240 = Bundle By Name(cluster=w780, "Z Stage.Position"=w782) -> (w784:T19)
                    n241 = flat-sequence {
                      tunnel: [w904] -> w791
                      tunnel: w794 -> [w903]
                      tunnel: w784 -> [w902]
                      frame #0 {
                        # "Go to Z0"
                        n242 = call "XYZ Table Stage Module.vi"("Set/Get"=Set_Get_Controls."Set", "Action"=Motion_Translation_Module_Control2."Position", "Error In"=w903, "Axis"=enum16{"X Axis", "Y Axis", "Z Axis"}."Z Axis", "Table Stages"=w902) -> ("Error Out"=w904:errorcluster)  [unwired: 5 in, 1 out]
                      }
                    }
                    n243 = Unbundle By Name(w772) -> ("Start X [mm]"=w792:dbl, "Start Y [mm]"=w793:dbl)
                    n244 = flat-sequence {
                      tunnel: w791 -> [w850]
                      tunnel: [w848] -> w790
                      tunnel: w789 -> [w847]
                      frame #0 {
                        # "Move to XY start"
                        n245 = call "XYZ Table Stage Module.vi"("Set/Get"=Set_Get_Controls."Set", "Action"=Motion_Translation_Module_Control2."Position", "Error In"=w850, "Axis"=enum16{"X Axis", "Y Axis", "Z Axis"}."X Axis", "Table Stages"=w847) -> ("Error Out"=w849:errorcluster, "Table Stages [out]"=w846:T19)  [unwired: 5 in]
                        n246 = call "XYZ Table Stage Module.vi"("Set/Get"=Set_Get_Controls."Set", "Action"=Motion_Translation_Module_Control2."Position", "Error In"=w849, "Axis"=enum16{"X Axis", "Y Axis", "Z Axis"}."Y Axis", "Table Stages"=w846) -> ("Error Out"=w848:errorcluster)  [unwired: 5 in, 1 out]
                      }
                    }
                    n247 = Bundle By Name(cluster=w780, "X Stage.Position"=w792, "Y Stage.Position"=w793) -> (w789:T19)
                    n248 = flat-sequence {
                      tunnel: [w892] -> w770
                      tunnel: w797 -> [w889]
                      tunnel: w790 -> [w890]
                      frame #0 {
                        # "Go to next cut height"
                        n249 = call "XYZ Table Stage Module.vi"("Set/Get"=Set_Get_Controls."Set", "Action"=Motion_Translation_Module_Control2."Position", "Error In"=w890, "Axis"=enum16{"X Axis", "Y Axis", "Z Axis"}."Z Axis", "Table Stages"=w889) -> ("Error Out"=w892:errorcluster)  [unwired: 5 in, 1 out]
                      }
                    }
                    n250 = Bundle By Name(cluster=w780, "Z Stage.Position"=w796) -> (w797:T19)
                    n251 = Array Size(array=w768) -> (size(s)=w767:i32)
                    n252 = Quotient & Remainder(x=w767, y=2) -> (x-y*floor(x/y)=w765:i32)  [unwired: 1 out]
                    n253 = case shown="\"every two slices\"" w764 {
                      tunnel: w765 -> [_ w804]
                      tunnel: w770 -> [w799 w802]
                      tunnel: [w799 w801] -> w771
                      frame "None", Default {
                      }
                      frame "every two slices" {
                        n254 = Equal?(x=w804, y=1) -> (x = y?=w800:bool)
                        n255 = case shown="True" w800 {
                          tunnel: w802 -> [w805 w819]
                          tunnel: [w805 w817] -> w801
                          frame False {
                          }
                          frame True {
                            n256 = call "Pause.vi"("action"=Pause_action."set", "error in"=w819, "Pause!"=TRUE) -> ("error out"=w818:errorcluster)  [unwired: 7 in, 1 out]
                            n257 = call "System Parameters - FGV.vi"("Actions"=FGV_Actions."Get", "Error In"=w818) -> ("Error Out"=w817:errorcluster, "System Parameters [Out]"=w815:T16)  [unwired: 8 in]
                            n258 = Unbundle By Name(w815) -> ("Manual Controls.Outgoing Mail Server (SMTP)"=w808:string, "Manual Controls.Email"=w812:string, "Manual Controls.Password"=w811:string, "Manual Controls.Carrier 1"=w814:enum16{"T-Mobile", "AT&T", "Verizon", "Sprint"}, "Manual Controls.phone number 1"=w813:string, "Manual Controls.Subject"=w810:string, "Manual Controls.Message"=w809:string, "Manual Controls.phone number 2"=w807:string, "Manual Controls.Carrier 2"=w806:enum16{"T-Mobile", "AT&T", "Verizon", "Sprint"})
                            n259 = call "Send Text Using SMTP API 2013 NIVerified.vi"("phone number 2"=w807, "Carrier 2"=w806, "Body"=w809, "Carrier 1"=w814, "Subject"=w810, "phone number 1"=w813, "Outgoing Mail Server (SMTP)"=w808, "Password"=w811, "Email"=w812) -> ()  [unwired: 3 in]
                          }
                        }
                      }
                    }
                    n260 = Unbundle By Name(w772) -> ("Start X [mm]"=w783:dbl, "Start Y [mm]"=w786:dbl, "Slice Length [mm]"=w785:dbl, "Slice Speed [mm/s]"=w787:dbl, "Slice Axis"=w788:enum16{"X Axis", "Y Axis", "Z Axis"}, "Ramp Time [s]"=w777:dbl)
                    n261 = flat-sequence {
                      tunnel: w769 -> [w841]
                      tunnel: [w833] -> w798
                      tunnel: [w845] -> w778
                      tunnel: w798 -> [w845]
                      tunnel: w777 -> [w843]
                      frame #0 {
                        n262 = call "vibratome3 module.vi"("Action"=vibratome3_control."Init", "error in"=w841) -> ("error out"=w836:errorcluster)  [unwired: 9 in]
                        n263 = call "vibratome3 module.vi"("Action"=vibratome3_control."Configure channel", "error in"=w836) -> ("error out"=w835:errorcluster)  [unwired: 9 in]
                        n264 = call "vibratome3 module.vi"("Action"=vibratome3_control."Write waveform", "error in"=w835) -> ("error out"=w834:errorcluster)  [unwired: 9 in]
                        n265 = call "vibratome3 module.vi"("Action"=vibratome3_control."Start", "error in"=w834) -> ("error out"=w833:errorcluster)  [unwired: 9 in]
                      }
                      frame #1 {
                        n266 = Multiply(x=w843, y=1000.0) -> (x*y=w844:dbl)
                        n267 = Wait (ms)(milliseconds to wait=w844) -> ()  [unwired: 1 out]
                      }
                    }
                    n268 = while {
                      tunnel: w771 -> [w825]
                      tunnel: [w822] -> w769
                      stop <- w826 stop-if-true
                      n269 = call "Pause.vi"("action"=Pause_action."get", "error in"=w825) -> ("error out"=w824:errorcluster, "Pause?"=w827:bool)  [unwired: 8 in]
                      n270 = Wait (ms)(milliseconds to wait=u32 200) -> ()  [unwired: 1 out]
                      n271 = case shown="False" w827 {
                        tunnel: [TRUE FALSE] -> w826
                        tunnel: w824 -> [w829 w831]
                        tunnel: [w829 w831] -> w822
                        frame False {
                        }
                        frame True {
                        }
                      }
                    }
                    n272 = case shown="\"X Axis\", Default" w788 {
                      tunnel: w787 -> [w864 w880]
                      tunnel: w778 -> [w863 w879]
                      tunnel: [w862 w878] -> w775
                      tunnel: w786 -> [w861 _]
                      tunnel: w785 -> [w860 w877]
                      tunnel: w780 -> [w858 w875]
                      tunnel: w783 -> [_ w873]
                      frame "Y Axis" {
                        n273 = Subtract(x=w861, y=w860) -> (x-y=w859:dbl)
                        n274 = Bundle By Name(cluster=w858, "Y Stage.Velocity"=w864, "Y Stage.Position"=w859) -> (w857:T19)
                        n275 = call "XYZ Table Stage Module.vi"("Set/Get"=Set_Get_Controls."Set", "Action"=Motion_Translation_Module_Control2."Velocity/Accel", "Error In"=w863, "Axis"=enum16{"X Axis", "Y Axis", "Z Axis"}."Y Axis", "Table Stages"=w857) -> ("Error Out"=w867:errorcluster, "Table Stages [out]"=w866:T19)  [unwired: 5 in]
                        n276 = call "XYZ Table Stage Module.vi"("Set/Get"=Set_Get_Controls."Set", "Action"=Motion_Translation_Module_Control2."Position", "Error In"=w867, "Axis"=enum16{"X Axis", "Y Axis", "Z Axis"}."Y Axis", "Table Stages"=w866) -> ("Error Out"=w862:errorcluster)  [unwired: 5 in, 1 out]
                      }
                      frame "X Axis", Default {
                        n277 = Subtract(x=w873, y=w877) -> (x-y=w876:dbl)
                        n278 = Bundle By Name(cluster=w875, "X Stage.Velocity"=w880, "X Stage.Position"=w876) -> (w874:T19)
                        n279 = call "XYZ Table Stage Module.vi"("Set/Get"=Set_Get_Controls."Set", "Action"=Motion_Translation_Module_Control2."Velocity/Accel", "Error In"=w879, "Axis"=enum16{"X Axis", "Y Axis", "Z Axis"}."X Axis", "Table Stages"=w874) -> ("Error Out"=w883:errorcluster, "Table Stages [out]"=w882:T19)  [unwired: 5 in]
                        n280 = call "XYZ Table Stage Module.vi"("Set/Get"=Set_Get_Controls."Set", "Action"=Motion_Translation_Module_Control2."Position", "Error In"=w883, "Axis"=enum16{"X Axis", "Y Axis", "Z Axis"}."X Axis", "Table Stages"=w882) -> ("Error Out"=w878:errorcluster)  [unwired: 5 in, 1 out]
                      }
                    }
                    n281 = call "vibratome3 module.vi"("Action"=vibratome3_control."Finish?", "error in"=w775) -> ("error out"=w774:errorcluster)  [unwired: 9 in]
                    n282 = call "vibratome3 module.vi"("Action"=vibratome3_control."Uninit", "error in"=w774) -> ("error out"=w773:errorcluster)  [unwired: 9 in]
                    n283 = Bundle By Name(cluster=w780, "Z Stage.Position"=w782) -> (w781:T19)
                    n284 = flat-sequence {
                      tunnel: [w898] -> w795
                      tunnel: w781 -> [w896]
                      tunnel: w773 -> [w895]
                      frame #0 {
                        # "Go to Z0"
                        n285 = call "XYZ Table Stage Module.vi"("Set/Get"=Set_Get_Controls."Set", "Action"=Motion_Translation_Module_Control2."Position", "Error In"=w895, "Axis"=enum16{"X Axis", "Y Axis", "Z Axis"}."Z Axis", "Table Stages"=w896) -> ("Error Out"=w898:errorcluster)  [unwired: 5 in, 1 out]
                      }
                    }
                  }
                  frame True {
                    (unwired) "Only works for 150um slices and 5x30um cuts"
                    n286 = flat-sequence {
                      tunnel: [w920] -> w908
                      tunnel: w910 -> [w919]
                      tunnel: w911 -> [w918]
                      frame #0 {
                        # "Go to Z0"
                        n287 = call "XYZ Table Stage Module.vi"("Set/Get"=Set_Get_Controls."Set", "Action"=Motion_Translation_Module_Control2."Position", "Error In"=w919, "Axis"=enum16{"X Axis", "Y Axis", "Z Axis"}."Z Axis", "Table Stages"=w918) -> ("Error Out"=w920:errorcluster)  [unwired: 5 in, 1 out]
                      }
                    }
                    n288 = Bundle By Name(cluster=w913, "Z Stage.Position"=w909) -> (w911:T19)
                    n289 = for {
                      N: 5 -> [_]
                      tunnel: w916 -> [w933]
                      shift-right: [w956] -> w915
                      shift-left: w908 -> [w928]
                      tunnel: w913 -> [w935]
                      tunnel: w912 -> [w934]
                      tunnel: w907 -> [w925]
                      i -> [w926]
                      n290 = Subtract(x=w933, y=0.12) -> (x-y=w931:dbl)
                      n291 = Unbundle By Name(w934) -> ("Start X [mm]"=w954:dbl, "Start Y [mm]"=w955:dbl)
                      n292 = flat-sequence {
                        tunnel: [w1009] -> w953
                        tunnel: w952 -> [w1008]
                        tunnel: w928 -> [w1006]
                        frame #0 {
                          # "Move to XY start"
                          n293 = call "XYZ Table Stage Module.vi"("Set/Get"=Set_Get_Controls."Set", "Action"=Motion_Translation_Module_Control2."Position", "Error In"=w1006, "Axis"=enum16{"X Axis", "Y Axis", "Z Axis"}."X Axis", "Table Stages"=w1008) -> ("Error Out"=w1010:errorcluster, "Table Stages [out]"=w1007:T19)  [unwired: 5 in]
                          n294 = call "XYZ Table Stage Module.vi"("Set/Get"=Set_Get_Controls."Set", "Action"=Motion_Translation_Module_Control2."Position", "Error In"=w1010, "Axis"=enum16{"X Axis", "Y Axis", "Z Axis"}."Y Axis", "Table Stages"=w1007) -> ("Error Out"=w1009:errorcluster)  [unwired: 5 in, 1 out]
                        }
                      }
                      n295 = Bundle By Name(cluster=w935, "X Stage.Position"=w954, "Y Stage.Position"=w955) -> (w952:T19)
                      n296 = Multiply(x=w926, y=0.03) -> (x*y=w937:dbl)
                      n297 = Add(x=w931, y=w937) -> (x+y=w936:dbl)
                      n298 = case shown="\"Nat slices\"" w925 {
                        tunnel: w926 -> [_ w964]
                        tunnel: w924 -> [w959 w961]
                        tunnel: [w959 w960] -> w927
                        frame "every two slices", Default {
                        }
                        frame "Nat slices" {
                          n299 = Equal?(x=w964, y=2) -> (x = y?=w962:bool)
                          n300 = case shown="True" w962 {
                            tunnel: w961 -> [w965 w979]
                            tunnel: [w965 w977] -> w960
                            frame False {
                            }
                            frame True {
                              n301 = call "Pause.vi"("action"=Pause_action."set", "error in"=w979, "Pause!"=TRUE) -> ("error out"=w978:errorcluster)  [unwired: 7 in, 1 out]
                              n302 = call "System Parameters - FGV.vi"("Actions"=FGV_Actions."Get", "Error In"=w978) -> ("Error Out"=w977:errorcluster, "System Parameters [Out]"=w975:T16)  [unwired: 8 in]
                              n303 = Unbundle By Name(w975) -> ("Manual Controls.Outgoing Mail Server (SMTP)"=w968:string, "Manual Controls.Email"=w972:string, "Manual Controls.Password"=w971:string, "Manual Controls.Carrier 1"=w974:enum16{"T-Mobile", "AT&T", "Verizon", "Sprint"}, "Manual Controls.phone number 1"=w973:string, "Manual Controls.Subject"=w970:string, "Manual Controls.Message"=w969:string, "Manual Controls.phone number 2"=w967:string, "Manual Controls.Carrier 2"=w966:enum16{"T-Mobile", "AT&T", "Verizon", "Sprint"})
                              n304 = call "Send Text Using SMTP API 2013 NIVerified.vi"("phone number 2"=w967, "Carrier 2"=w966, "Body"=w969, "Carrier 1"=w974, "Subject"=w970, "phone number 1"=w973, "Outgoing Mail Server (SMTP)"=w968, "Password"=w971, "Email"=w972) -> ()  [unwired: 3 in]
                            }
                          }
                        }
                      }
                      n305 = flat-sequence {
                        tunnel: [w1052] -> w924
                        tunnel: w957 -> [w1049]
                        tunnel: w953 -> [w1050]
                        frame #0 {
                          # "Go to next cut height"
                          n306 = call "XYZ Table Stage Module.vi"("Set/Get"=Set_Get_Controls."Set", "Action"=Motion_Translation_Module_Control2."Position", "Error In"=w1050, "Axis"=enum16{"X Axis", "Y Axis", "Z Axis"}."Z Axis", "Table Stages"=w1049) -> ("Error Out"=w1052:errorcluster)  [unwired: 5 in, 1 out]
                        }
                      }
                      n307 = Bundle By Name(cluster=w935, "Z Stage.Position"=w936) -> (w957:T19)
                      n308 = flat-sequence {
                        tunnel: w923 -> [w1001]
                        tunnel: [w993] -> w958
                        tunnel: [w1005] -> w944
                        tunnel: w958 -> [w1005]
                        tunnel: w943 -> [w1003]
                        frame #0 {
                          n309 = call "vibratome3 module.vi"("Action"=vibratome3_control."Init", "error in"=w1001) -> ("error out"=w996:errorcluster)  [unwired: 9 in]
                          n310 = call "vibratome3 module.vi"("Action"=vibratome3_control."Configure channel", "error in"=w996) -> ("error out"=w995:errorcluster)  [unwired: 9 in]
                          n311 = call "vibratome3 module.vi"("Action"=vibratome3_control."Write waveform", "error in"=w995) -> ("error out"=w994:errorcluster)  [unwired: 9 in]
                          n312 = call "vibratome3 module.vi"("Action"=vibratome3_control."Start", "error in"=w994) -> ("error out"=w993:errorcluster)  [unwired: 9 in]
                        }
                        frame #1 {
                          n313 = Multiply(x=w1003, y=1000.0) -> (x*y=w1004:dbl)
                          n314 = Wait (ms)(milliseconds to wait=w1004) -> ()  [unwired: 1 out]
                        }
                      }
                      n315 = Unbundle By Name(w934) -> ("Start X [mm]"=w947:dbl, "Start Y [mm]"=w949:dbl, "Slice Length [mm]"=w948:dbl, "Slice Speed [mm/s]"=w950:dbl, "Slice Axis"=w951:enum16{"X Axis", "Y Axis", "Z Axis"}, "Ramp Time [s]"=w943:dbl)
                      n316 = while {
                        tunnel: w927 -> [w985]
                        tunnel: [w983] -> w923
                        stop <- w986 stop-if-true
                        n317 = call "Pause.vi"("action"=Pause_action."get", "error in"=w985) -> ("error out"=w984:errorcluster, "Pause?"=w987:bool)  [unwired: 8 in]
                        n318 = Wait (ms)(milliseconds to wait=u32 200) -> ()  [unwired: 1 out]
                        n319 = case shown="False" w987 {
                          tunnel: [TRUE FALSE] -> w986
                          tunnel: w984 -> [w989 w991]
                          tunnel: [w989 w991] -> w983
                          frame False {
                          }
                          frame True {
                          }
                        }
                      }
                      n320 = case shown="\"X Axis\", Default" w951 {
                        tunnel: w950 -> [w1024 w1040]
                        tunnel: w944 -> [w1023 w1039]
                        tunnel: [w1022 w1038] -> w941
                        tunnel: w949 -> [w1021 _]
                        tunnel: w948 -> [w1020 w1037]
                        tunnel: w935 -> [w1018 w1035]
                        tunnel: w947 -> [_ w1033]
                        frame "Y Axis" {
                          n321 = Subtract(x=w1021, y=w1020) -> (x-y=w1019:dbl)
                          n322 = Bundle By Name(cluster=w1018, "Y Stage.Velocity"=w1024, "Y Stage.Position"=w1019) -> (w1017:T19)
                          n323 = call "XYZ Table Stage Module.vi"("Set/Get"=Set_Get_Controls."Set", "Action"=Motion_Translation_Module_Control2."Velocity/Accel", "Error In"=w1023, "Axis"=enum16{"X Axis", "Y Axis", "Z Axis"}."Y Axis", "Table Stages"=w1017) -> ("Error Out"=w1027:errorcluster, "Table Stages [out]"=w1026:T19)  [unwired: 5 in]
                          n324 = call "XYZ Table Stage Module.vi"("Set/Get"=Set_Get_Controls."Set", "Action"=Motion_Translation_Module_Control2."Position", "Error In"=w1027, "Axis"=enum16{"X Axis", "Y Axis", "Z Axis"}."Y Axis", "Table Stages"=w1026) -> ("Error Out"=w1022:errorcluster)  [unwired: 5 in, 1 out]
                        }
                        frame "X Axis", Default {
                          n325 = Subtract(x=w1033, y=w1037) -> (x-y=w1036:dbl)
                          n326 = Bundle By Name(cluster=w1035, "X Stage.Velocity"=w1040, "X Stage.Position"=w1036) -> (w1034:T19)
                          n327 = call "XYZ Table Stage Module.vi"("Set/Get"=Set_Get_Controls."Set", "Action"=Motion_Translation_Module_Control2."Velocity/Accel", "Error In"=w1039, "Axis"=enum16{"X Axis", "Y Axis", "Z Axis"}."X Axis", "Table Stages"=w1034) -> ("Error Out"=w1043:errorcluster, "Table Stages [out]"=w1042:T19)  [unwired: 5 in]
                          n328 = call "XYZ Table Stage Module.vi"("Set/Get"=Set_Get_Controls."Set", "Action"=Motion_Translation_Module_Control2."Position", "Error In"=w1043, "Axis"=enum16{"X Axis", "Y Axis", "Z Axis"}."X Axis", "Table Stages"=w1042) -> ("Error Out"=w1038:errorcluster)  [unwired: 5 in, 1 out]
                        }
                      }
                      n329 = call "vibratome3 module.vi"("Action"=vibratome3_control."Finish?", "error in"=w941) -> ("error out"=w940:errorcluster)  [unwired: 9 in]
                      n330 = Subtract(x=w931, y=0.1) -> (x-y=w929:dbl)
                      n331 = call "vibratome3 module.vi"("Action"=vibratome3_control."Uninit", "error in"=w940) -> ("error out"=w939:errorcluster)  [unwired: 9 in]
                      n332 = Bundle By Name(cluster=w935, "Z Stage.Position"=w929) -> (w946:T19)
                      n333 = flat-sequence {
                        tunnel: [w1057] -> w956
                        tunnel: w946 -> [w1055]
                        tunnel: w939 -> [w1061]
                        frame #0 {
                          # "Go to Z0"
                          n334 = call "XYZ Table Stage Module.vi"("Set/Get"=Set_Get_Controls."Set", "Action"=Motion_Translation_Module_Control2."Position", "Error In"=w1061, "Axis"=enum16{"X Axis", "Y Axis", "Z Axis"}."Z Axis", "Table Stages"=w1055) -> ("Error Out"=w1058:errorcluster)  [unwired: 5 in, 1 out]
                          n335 = call "XYZ Table Stage Module.vi"("Set/Get"=Set_Get_Controls."Set", "Action"=Motion_Translation_Module_Control2."Velocity/Accel", "Error In"=w1058, "Axis"=enum16{"X Axis", "Y Axis", "Z Axis"}."X Axis", "Table Stages"=w1055) -> ("Error Out"=w1057:errorcluster)  [unwired: 5 in, 1 out]
                        }
                      }
                    }
                  }
                }
              }
            }
            n336 = call "System Parameters - FGV.vi"("Actions"=FGV_Actions."Get") -> ("System Parameters [Out]"=w728:T16)  [unwired: 9 in, 1 out]
            n337 = Unbundle By Name(w728) -> ("Vibratome Axis.#images"=w740:u16)
            n338 = for {
              N: w740 -> [_]
              shift-right: [w1066] -> w737
              shift-left: w739 -> [w1065]
              w1067 = T1[] [enum."Generate Mosaic", enum."Go Image Home", enum."Go to Image Z", enum."Go Mosaic", enum."Init Scan Head"] items=["Init(ThorOCT Spatial)", "Init(ThorOCT Spectral)", "Init(GPU FFT)", "Init(Alazar FFT)", "Init Scan Head(ThorOCT Spectral)", "Init Scan Head(ThorOCT Spatial)", "Init Scan Head", "Init Table Stage", "Init Vibratome", "Generate Mosaic", "Generate Z Position", "Go to Image Z", "Go Image Home", "Go Mosaic", "Acquire Image(ThorOCT Spatial)", "Acquire Image(ThorOCT Spectral)", "Acquire Image(GPU FFT)", "Acquire Image(Alazar FFT)", "Go Vibratome", "Slice", "Finished(ThorOCT)", "Finished", "Init(Alazar Spectral)", "Go Vibratome3"]
              n339 = Build Array (concatenate)(w1065, w1067) -> (w1066:T1[])
            }
            n340 = Build Array (concatenate)(w737, w736, w738) -> (w745:T1[])
          }
          frame True {
          }
        }
      }
      frame "Slice" {
        n341 = case shown="False" FALSE {
          tunnel: w1091 -> [w1100 w1111]
          tunnel: [w1100 w1111] -> w1089
          tunnel: [w1101 w1110] -> w1090
          tunnel: w1088 -> [w1097 w1110]
          frame False {
            n342 = call "System Parameters - FGV.vi"("Actions"=FGV_Actions."Get", "Error In"=w1097) -> ("Error Out"=w1096:errorcluster, "System Parameters [Out]"=w1095:T16)  [unwired: 8 in]
            n343 = Unbundle By Name(w1095) -> ("Table Stages"=w1103:T19, "Vibratome"=w1099:T18, "Vibratome.Blade Frequency [Hz]"=w1094:u16)
            n344 = call "Slice Engine.vi"("Table Stages"=w1103, "error in (no error)"=w1096, "Vibratome"=w1099, "Action"="Move Stage (XY)") -> ("error out"=w1102:errorcluster)  [unwired: 7 in]
            n345 = call "Slice Engine.vi"("Table Stages"=w1103, "error in (no error)"=w1102, "Vibratome"=w1099, "Action"="Set Slice Speed") -> ("error out"=w1104:errorcluster)  [unwired: 7 in]
            n346 = Not Equal To 0?(x=w1094) -> (x != 0?=w1093:bool)
            n347 = case shown="False" w1093 {
              tunnel: ["Slice" ("Action") "Slice3" ("Action")] -> w1105
              frame False {
              }
              frame True {
              }
            }
            n348 = call "Slice Engine.vi"("Table Stages"=w1103, "error in (no error)"=w1104, "Vibratome"=w1099, "Action"=w1105) -> ("error out"=w1101:errorcluster)  [unwired: 7 in]
          }
          frame True {
          }
        }
        n349 = Empty Array?(array=w1084) -> (empty?=w1085:bool)
      }
      frame "Finished", Default {
        n350 = call "Slice Engine.vi"("error in (no error)"=w1115, "Action"="Uninit") -> ("error out"=w1117:errorcluster)  [unwired: 9 in]
        n351 = call "Image Acquiring Module.vi"("Scan Status in"=scan_status."Finish Scan(PSOCT)", "Error in"=w1117) -> ("Error Out"=w1124:errorcluster)  [unwired: 9 in]
        n352 = call "FGV - Acquisition Status.vi"("Actions"=FGV_Actions."Get", "Error In"=w1124) -> ("Error Out"=w1125:errorcluster, "Quit status out"=w1120:bool, "Scan Type [Out]"=w1121:T15, "mem loc out"=w1119:i32)  [unwired: 6 in]
        n353 = call "FGV - Acquisition Status.vi"("mem loc"=w1119, "Actions"=FGV_Actions."Set", "Error In"=w1125, "Quit status"=w1120, "Scan Type [In]"=w1121) -> ("Error Out"=w1114:errorcluster)  [unwired: 3 in, 3 out]
        n354 = disable-structure shown="Enabled" {
          disable-tunnel: w1114 -> [w1128 w1131]
          disable-tunnel: [w1127 w1131] -> w1113
          frame Enabled {
            n355 = flat-sequence {
              tunnel: w1128 -> [w1130]
              tunnel: [w1130] -> w1127
              frame #0 {
                n356 = Wait (ms)(milliseconds to wait=u32 5000) -> ()  [unwired: 1 out]
              }
            }
          }
          frame Disabled {
          }
        }
        n357 = disable-structure shown="Enabled" {
          disable-tunnel: [w1135 w1137] -> w1112
          disable-tunnel: w1113 -> [w1132 w1137]
          frame Enabled {
            n358 = call "Save bline to memory1.vi"("action"=Save_Bline_to_Mem_Control."Uninit", "error in"=w1132) -> ("error out"=w1136:errorcluster)  [unwired: 13 in]
            n359 = call "Save bline to memory2.vi"("action"=Save_Bline_to_Mem_Control."Uninit", "error in"=w1136) -> ("error out"=w1135:errorcluster)  [unwired: 13 in]
          }
          frame Disabled {
          }
        }
      }
    }
  }
  n360 = call "Error Message Handler.vi"("Error In"=w9) -> ("Error Out"=→"Error Out":errorcluster, "T button?"=w7:bool)  [unwired: 9 in]
  n361 = Or(x=w6, y=w7) -> (x .or. y?=→"Finished?":bool)
